vi "Calibration.vi"(7 "Show Front Panel":bool=TRUE, 8 "error in (no error)":errorcluster, 11 "file path (dialog if empty)":path=path "C:/Program Files/GE/Washer DOE/CalibrationDates.txt") -> (0 "error out":errorcluster, 3 "OutputData":string[][](array[string]))   [LabVIEW 2012]
uses:
  Calibration.ctl
  CalibrationTime.ctl
  Calibration_SN.ctl
  Equipment.vi
  <vilib>/Utility/file.llb/Write To Spreadsheet File (string).vi
panel:
  in  "Size":i32
  out "snta":string[](array[string])
  in  "Tab Control":enum32{"Calibration Dates", "File Location"}(tab)
  in  "Equipment Description":T1
  in  "Manufacturer":T1
  in  "Model Number":T1
  in  "Calibration ID":T1
  in  "Complete":bool
  out "concatenated string":string
  in  "Serial Number":T2
  in  "Last Calibrated":T3 {"Eq20" format="%<%x>T"; "Eq19" format="%<%x>T"; "Eq18" format="%<%x>T"; "Eq17" format="%<%x>T"; "Eq16" format="%<%x>T"; "Eq15" format="%<%x>T"; "Eq14" format="%<%x>T"; "Eq13" format="%<%x>T"; "Eq12" format="%<%x>T"; "Eq11" format="%<%x>T"; "Eq10" format="%<%x>T"; "Eq9" format="%<%x>T"; "Eq8" format="%<%x>T"; "Eq7" format="%<%x>T"; "Eq6" format="%<%x>T"; "Eq5" format="%<%x>T"; "Eq4" format="%<%x>T"; "Eq3" format="%<%x>T"; "Eq2" format="%<%x>T"; "Eq1" format="%<%x>T"}
  in  "Calibration Due":T3 {"Eq20" format="%<%x>T"; "Eq19" format="%<%x>T"; "Eq18" format="%<%x>T"; "Eq17" format="%<%x>T"; "Eq16" format="%<%x>T"; "Eq15" format="%<%x>T"; "Eq14" format="%<%x>T"; "Eq13" format="%<%x>T"; "Eq12" format="%<%x>T"; "Eq11" format="%<%x>T"; "Eq10" format="%<%x>T"; "Eq9" format="%<%x>T"; "Eq8" format="%<%x>T"; "Eq7" format="%<%x>T"; "Eq6" format="%<%x>T"; "Eq5" format="%<%x>T"; "Eq4" format="%<%x>T"; "Eq3" format="%<%x>T"; "Eq2" format="%<%x>T"; "Eq1" format="%<%x>T"}
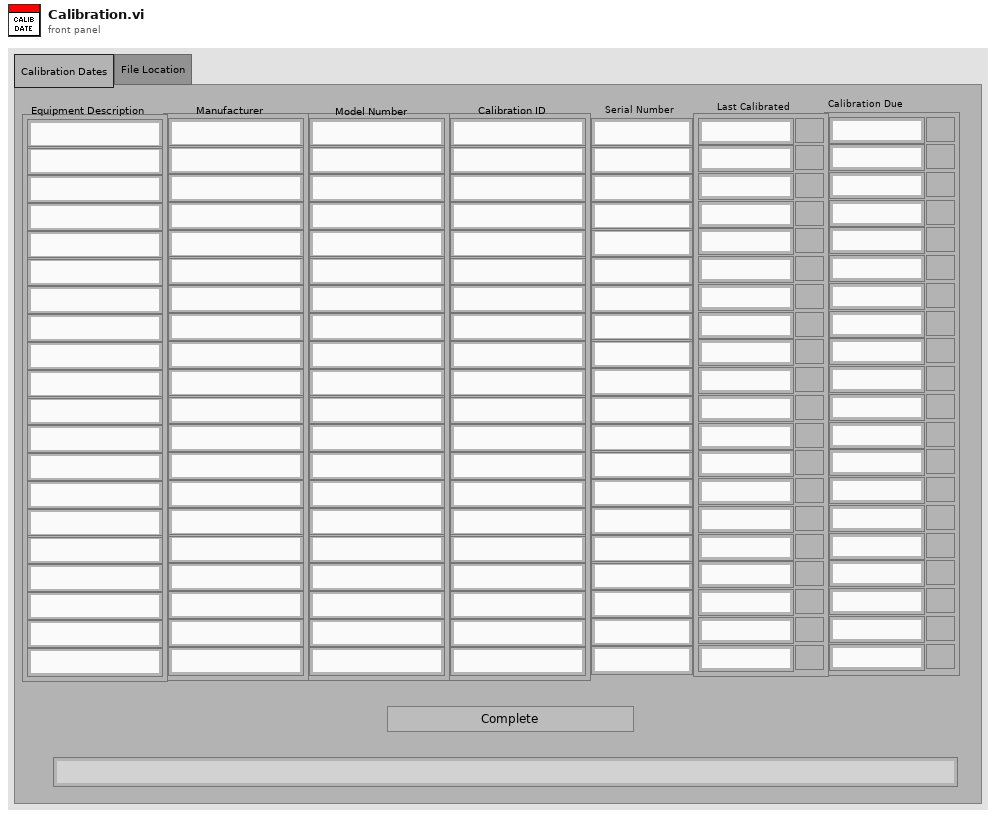
[diagram p1: front panel]
types:
  T1 = typedef "Calibration.ctl" = cluster{"Eq1":string, "Eq2":string, "Eq3":string, "Eq4":string, "Eq5":string, "Eq6":string, "Eq7":string, "Eq8":string, "Eq9":string, "Eq10":string, "Eq11":string, "Eq12":string, "Eq13":string, "Eq14":string, "Eq15":string, "Eq16":string, "Eq17":string, "Eq18":string, "Eq19":string, "Eq20":string}
  T2 = typedef "Calibration_SN.ctl" = cluster{"Eq1":string, "Eq2":string, "Eq3":string, "Eq4":string, "Eq5":string, "Eq6":string, "Eq7":string, "Eq8":string, "Eq9":string, "Eq10":string, "Eq11":string, "Eq12":string, "Eq13":string, "Eq14":string, "Eq15":string, "Eq16":string, "Eq17":string, "Eq18":string, "Eq19":string, "Eq20":string}
  T3 = typedef "CalibrationTime.ctl" = cluster{"Eq1":timestamp, "Eq2":timestamp, "Eq3":timestamp, "Eq4":timestamp, "Eq5":timestamp, "Eq6":timestamp, "Eq7":timestamp, "Eq8":timestamp, "Eq9":timestamp, "Eq10":timestamp, "Eq11":timestamp, "Eq12":timestamp, "Eq13":timestamp, "Eq14":timestamp, "Eq15":timestamp, "Eq16":timestamp, "Eq17":timestamp, "Eq18":timestamp, "Eq19":timestamp, "Eq20":timestamp}
  T4 = cluster{"Calibration Due":T3, "Last Calibrated":T3, "Serial Number":T2, "Calibration ID":T1, "Model Number":T1, "Manufacturer":T1, "Equipment Description":T1, i32}
  T5 = enum32{"invalid app kind", "Development System", "Run Time System", "Student Edition", "Embedded LabVIEW", "Evaluation", "Custom"}
  T6 = enum32{"Invalid", "Standard", "Closed", "Hidden", "Minimized", "Maximized"}
  T7 = cluster{"Core":cluster{"Current VI Reference":refnum<vi>, "Close Panel on Exit?":bool}, "Calibration Due":T3, "file path (dialog if empty)":path, "Serial Number":T2, "Calibration ID":T1, "Total Array":string[][], "Size":i32, "Last Calibrated":T3, "Model Number":T1, "Manufacturer":T1, "Equipment Description":T1}
  T8 = cluster{"Current VI Reference":refnum<vi>, "Close Panel on Exit?":bool}
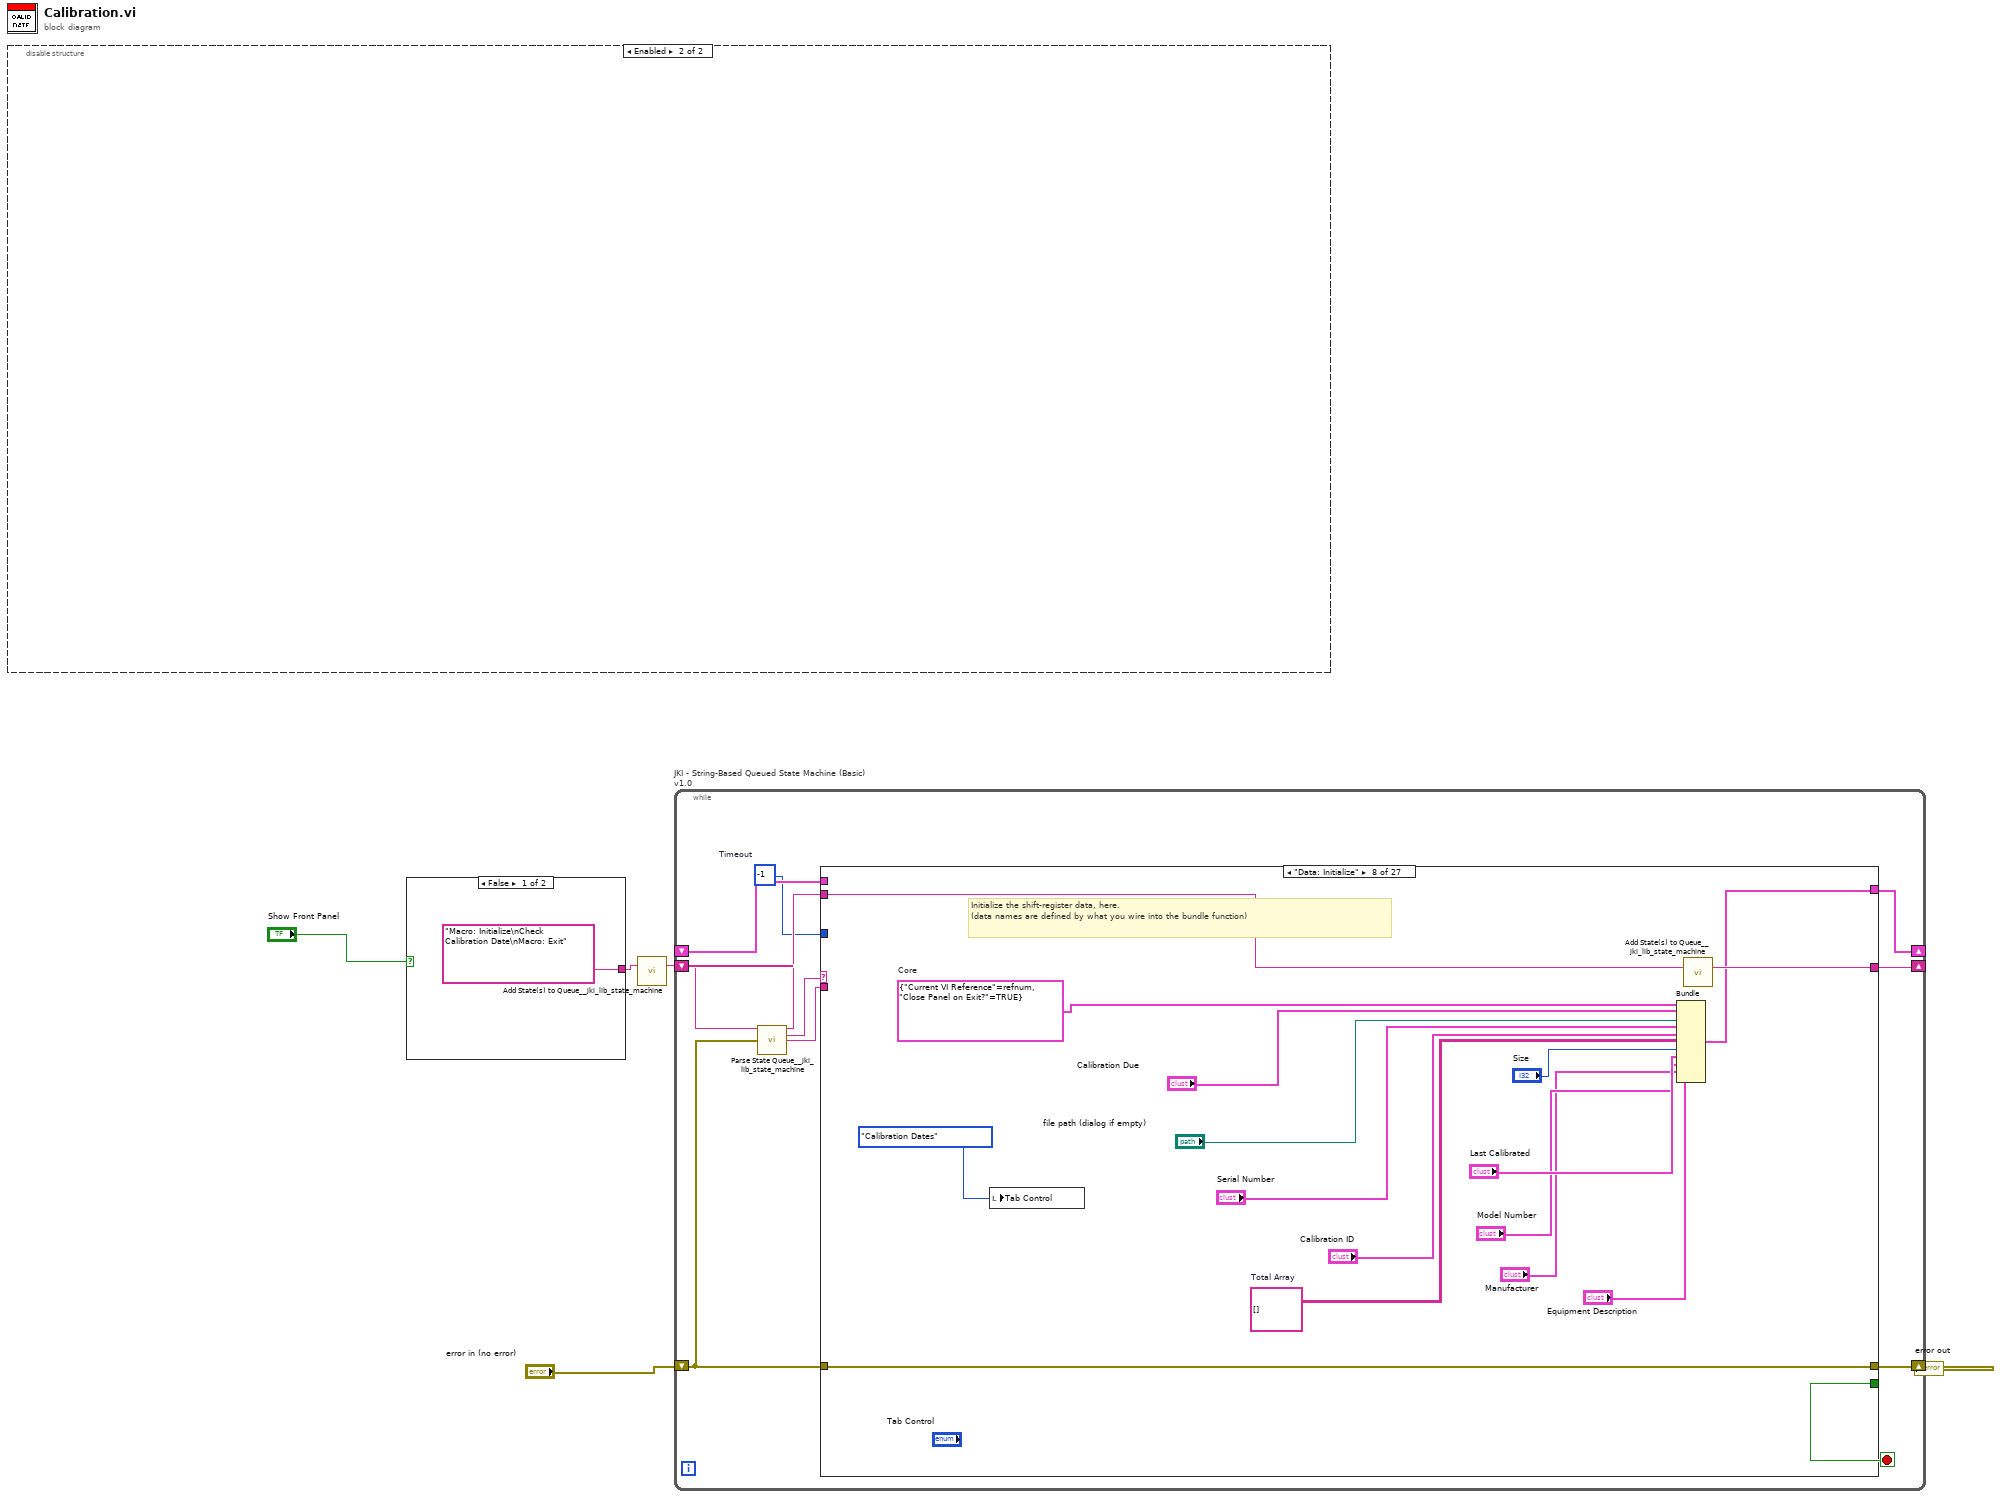
[diagram p0: block diagram]
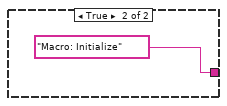
[diagram p2: hidden frame]
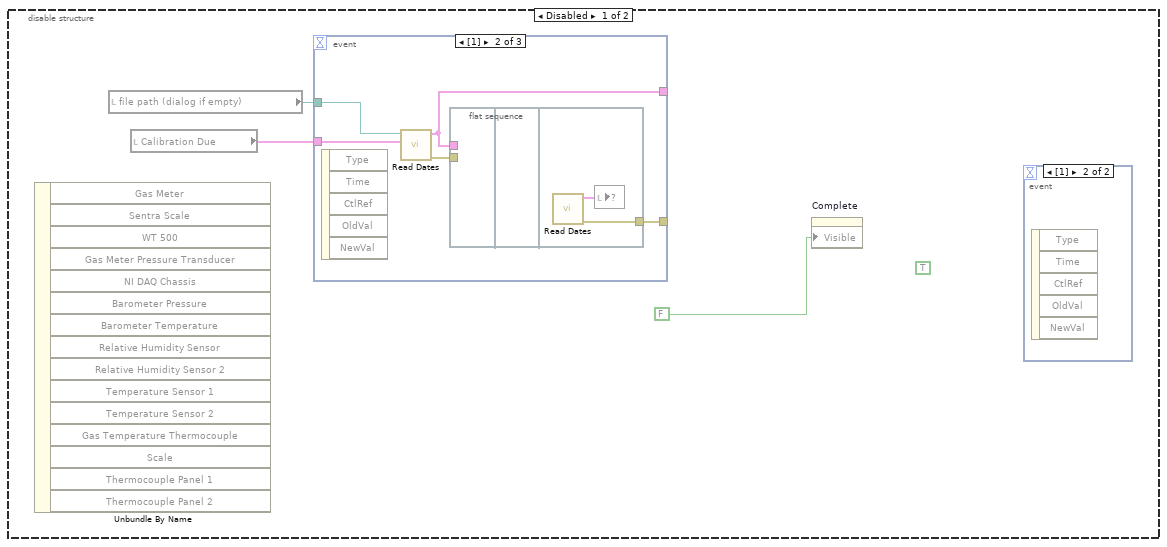
[diagram p3: hidden frame]
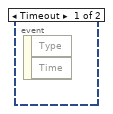
[diagram p4: hidden frame]
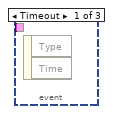
[diagram p5: hidden frame]
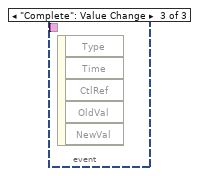
[diagram p6: hidden frame]
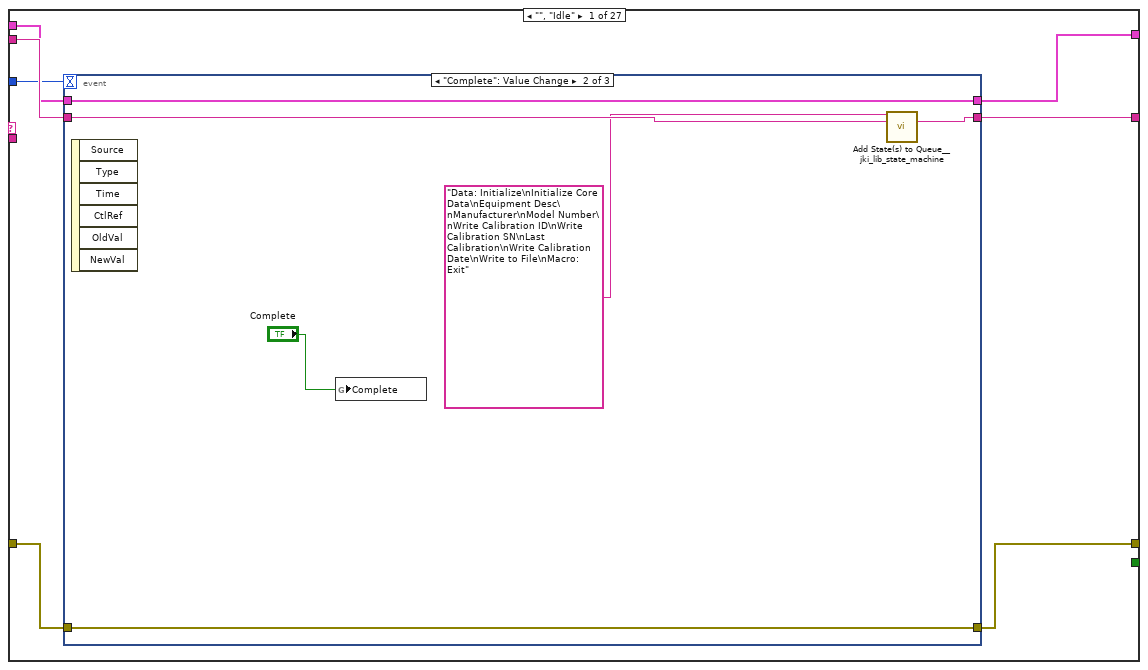
[diagram p7: hidden frame]
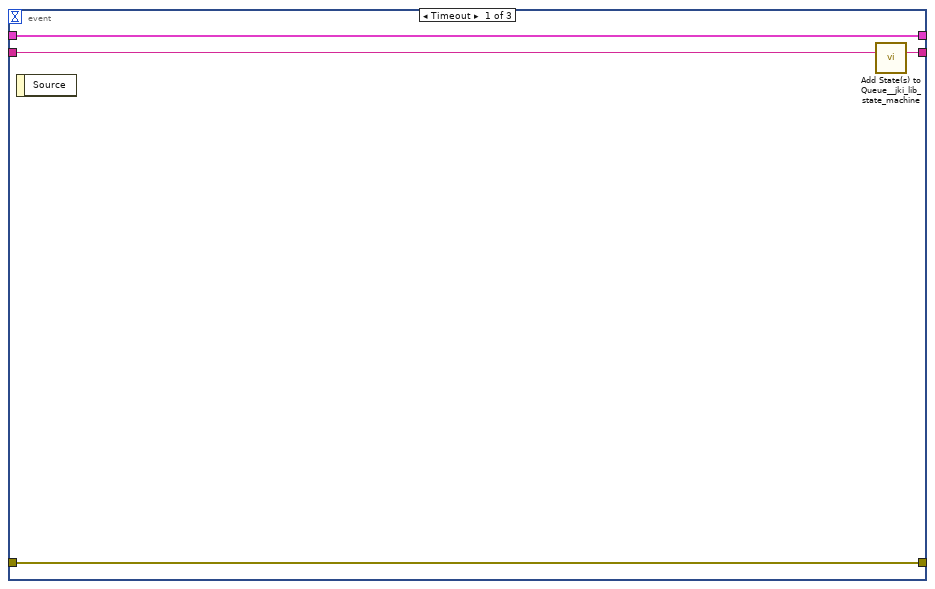
[diagram p8: hidden frame]
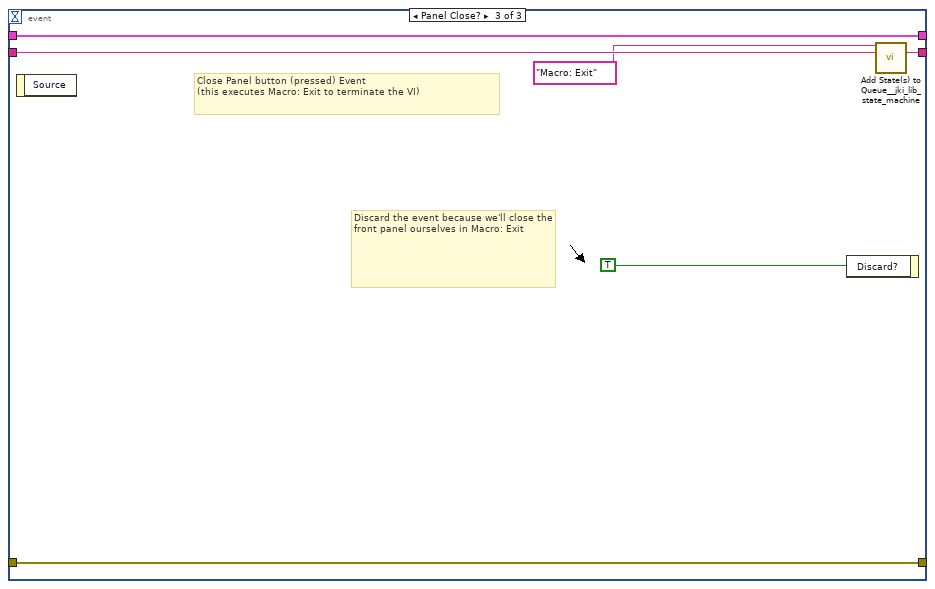
[diagram p9: hidden frame]
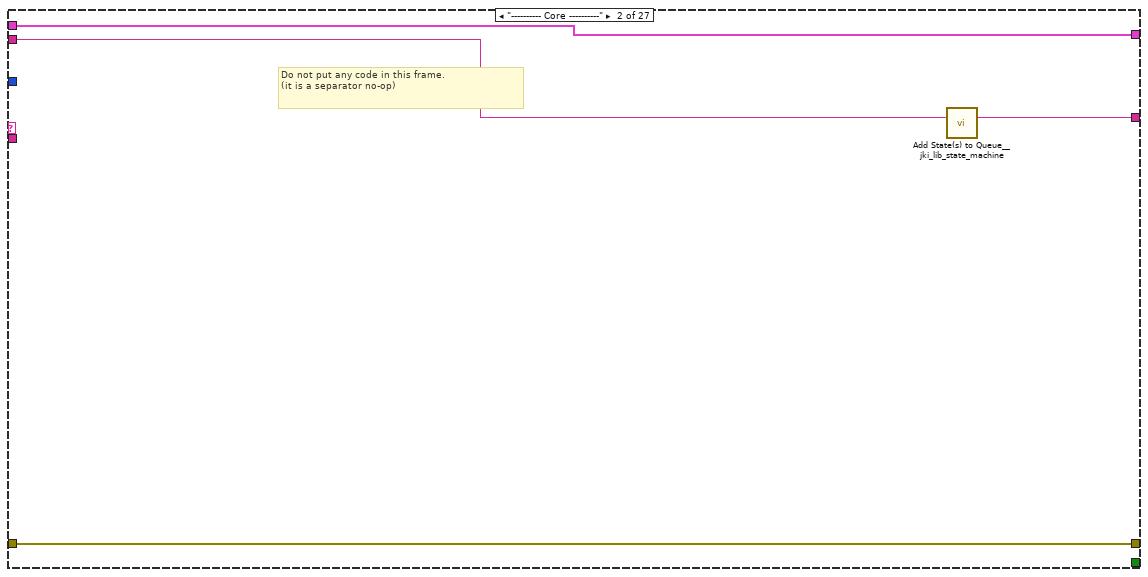
[diagram p10: hidden frame]
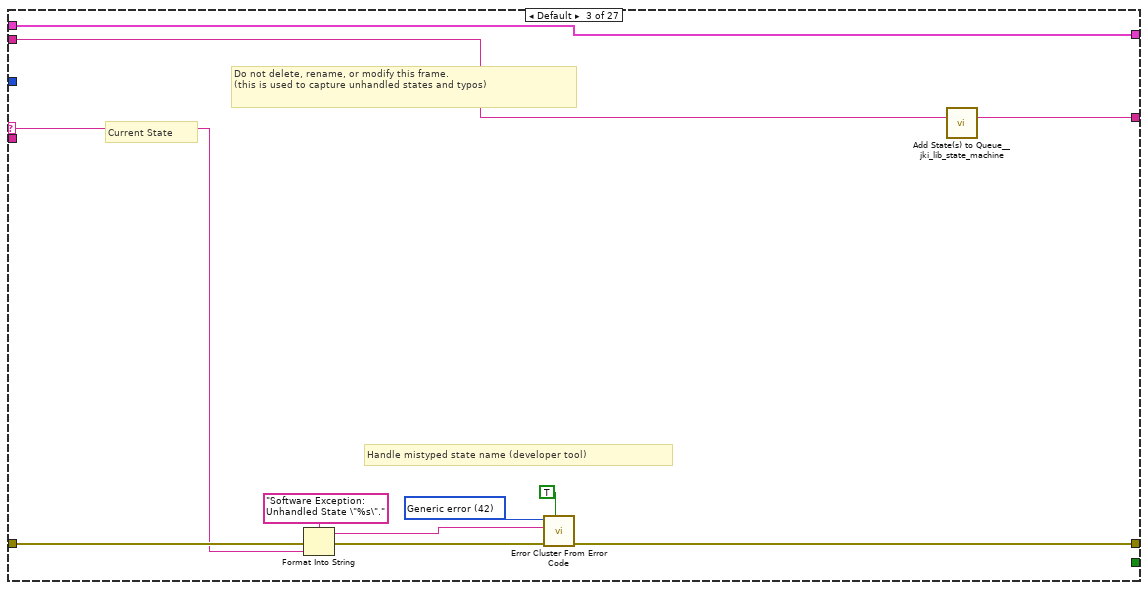
[diagram p11: hidden frame]
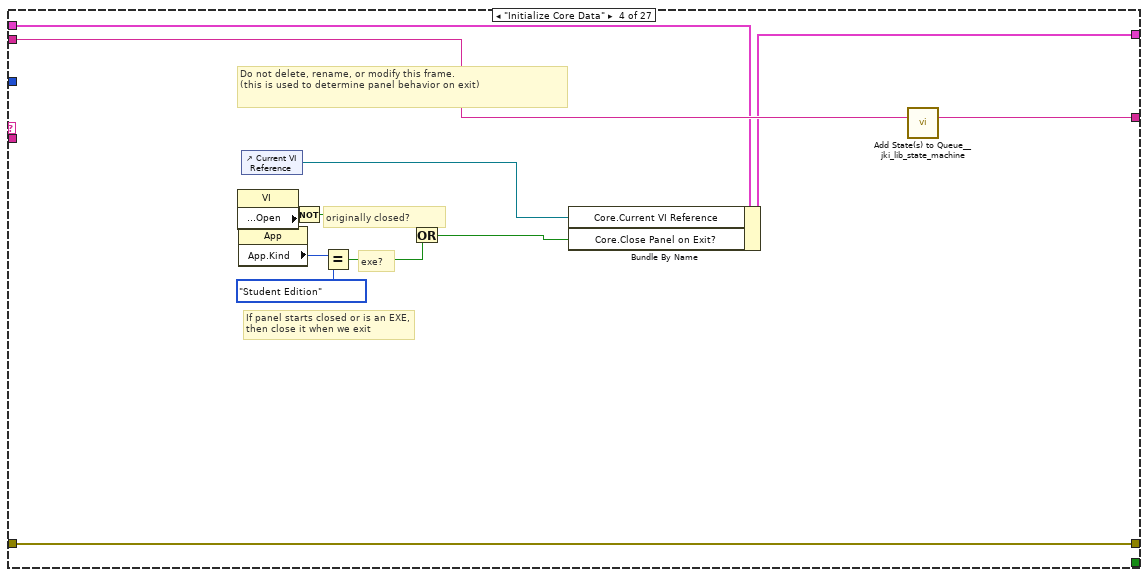
[diagram p12: hidden frame]
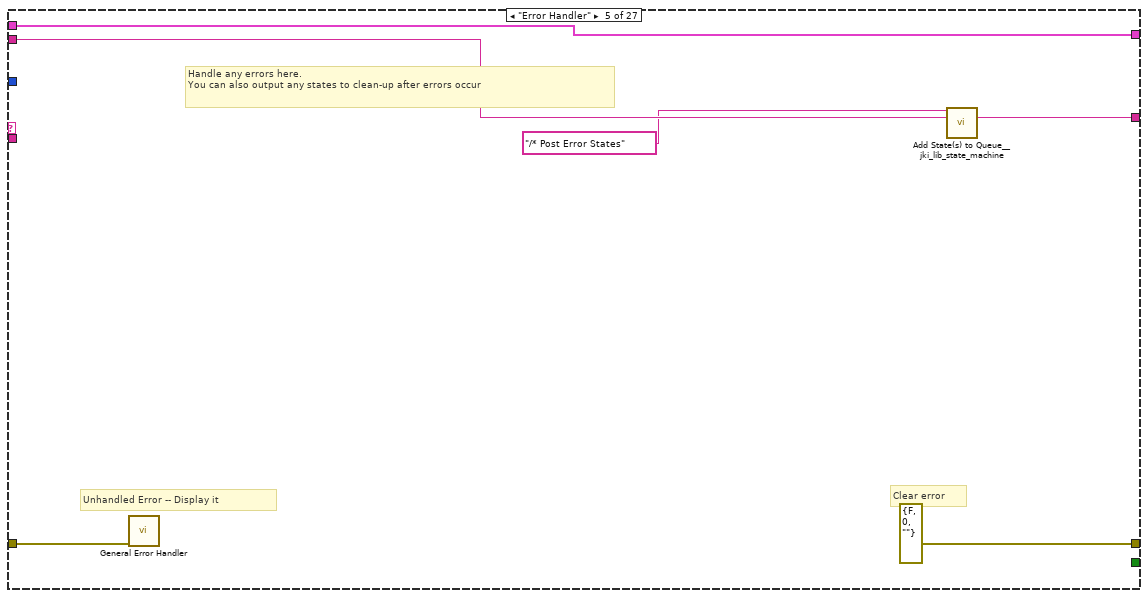
[diagram p13: hidden frame]
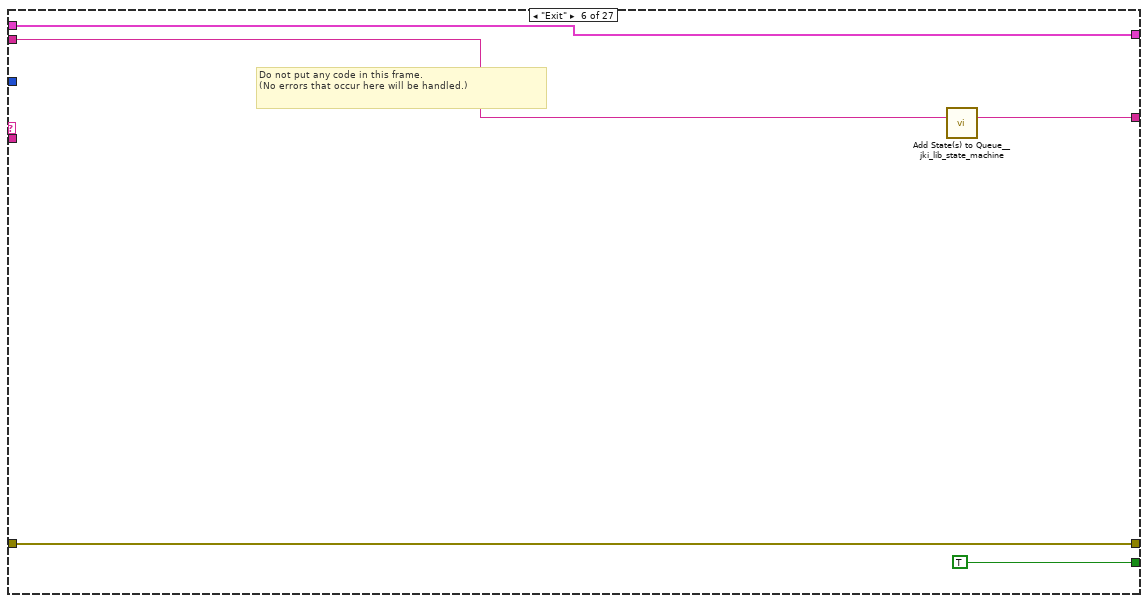
[diagram p14: hidden frame]
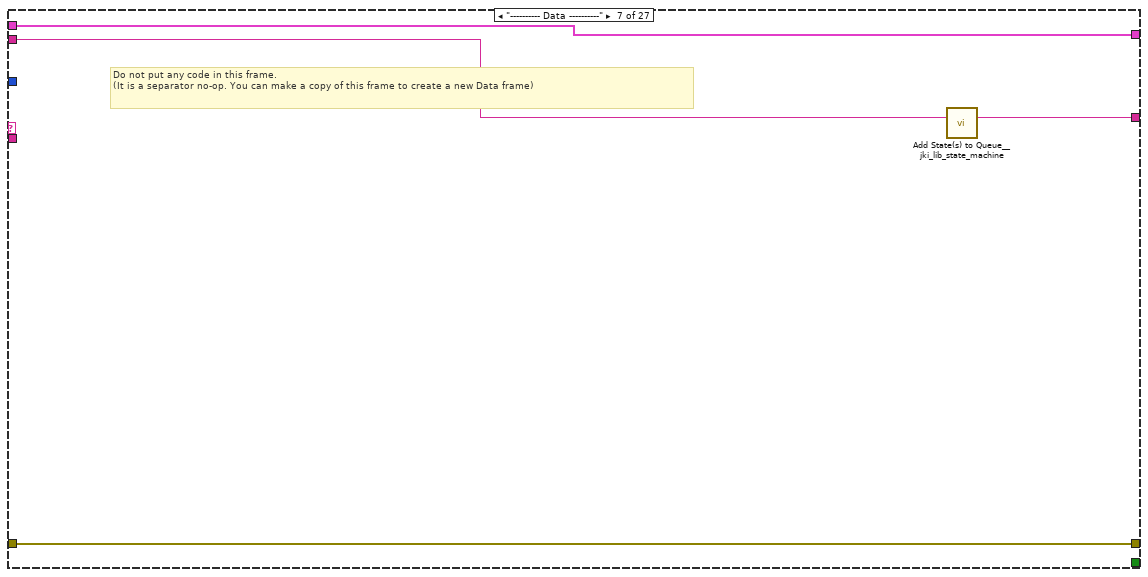
[diagram p15: hidden frame]
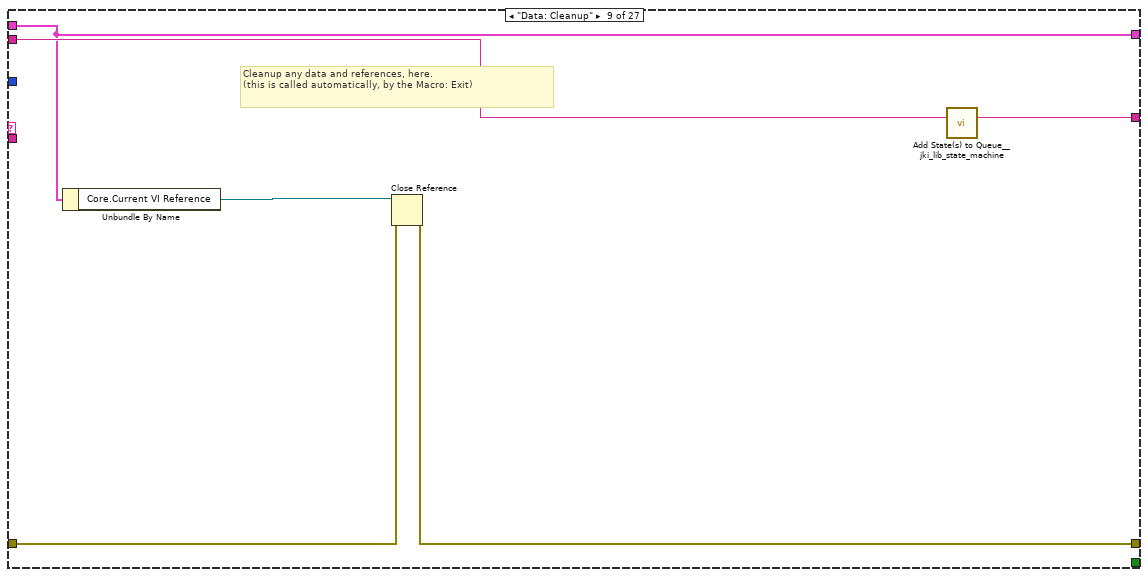
[diagram p16: hidden frame]
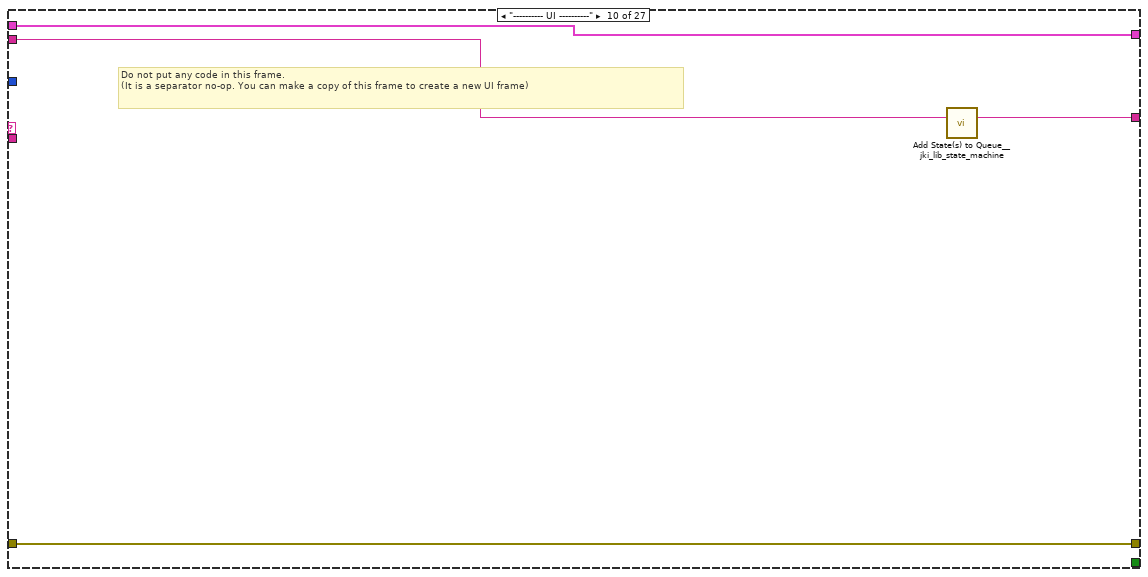
[diagram p17: hidden frame]
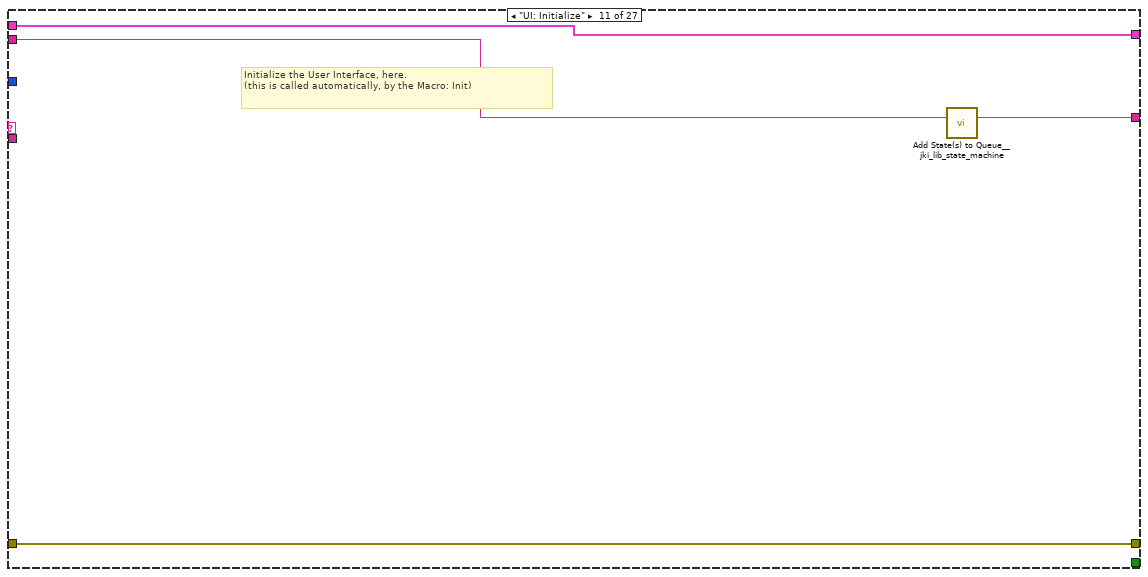
[diagram p18: hidden frame]
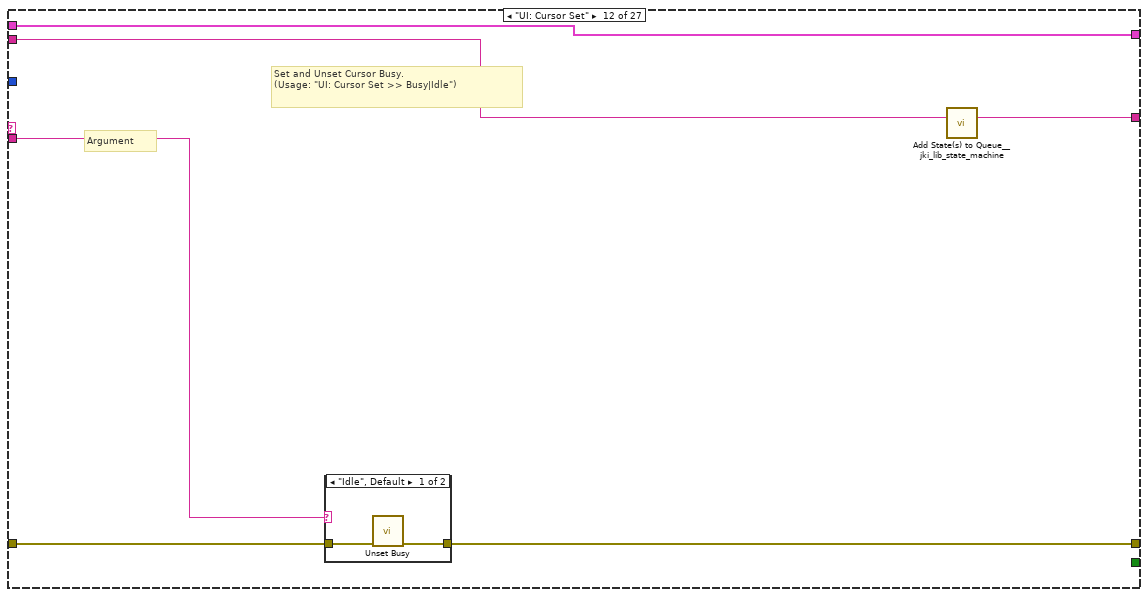
[diagram p19: hidden frame]
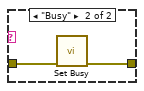
[diagram p20: hidden frame]
diagram:
  n1 = disable-structure shown="Enabled" {
    frame Disabled {
      w8 = TRUE ("Visible")
      n2 = Unbundle By Name() -> ()  [unwired: 1 in, 15 out]
      n3 = local read "file path (dialog if empty)"() -> (w6:path)
      n4 = local read "Calibration Due"() -> (w7:T3)
      n5 = event shown="[1]" {
        selector: _ -> [_ _ _]
        dyn-events: _ -> [_ _ _]
        timeout: _ -> [_ _ _]
        tunnel: [_ w12 _] -> _
        tunnel: [_ w15 _] -> _
        tunnel: w7 -> [_ w14 _]
        tunnel: w6 -> [_ w13 _]
        event Timeout {
          n6 = event-data() -> ()  [unwired: 1 in, 2 out]
        }
        event #1 (no event record) {
          n7 = event-data() -> ()  [unwired: 1 in, 5 out]
          n8 = call "Read Dates.vi"("Manufacturer"=w14, "Equipment Description"=w13) -> ("error out"=w11:errorcluster, "output cluster"=w12:T4)  [unwired: 8 in]
          n9 = flat-sequence {
            tunnel: w11 -> [_]
            tunnel: w12 -> [_]
            tunnel: [w16] -> w15
            frame #0 {
            }
            frame #1 {
            }
            frame #2 {
              n10 = call "Read Dates.vi"() -> ("error out"=w16:errorcluster, "output cluster"=w17:T4)  [unwired: 10 in]
              n11 = local write item#-1(w17) -> ()
            }
          }
        }
        event "Complete": Value Change {
          n12 = event-data() -> ()  [unwired: 1 in, 5 out]
        }
      }
      n13 = property on="Complete" class="Bool"("Visible"=FALSE) -> (error out=w9:errorcluster)  [unwired: 2 in, 1 out]
      n14 = event shown="[1]" {
        selector: _ -> [_ _]
        dyn-events: _ -> [_ _]
        timeout: _ -> [_ _]
        event Timeout {
          n15 = event-data() -> ()  [unwired: 1 in, 2 out]
        }
        event #1 (no event record) {
          n16 = event-data() -> ()  [unwired: 1 in, 5 out]
        }
      }
    }
    frame Enabled {
    }
  }
  n17 = case shown="False" "Show Front Panel" {
    tunnel: ["Macro: Initialize\nCheck Calibration Date\nMacro: Exit" "Macro: Initialize"] -> w4
    frame False {
    }
    frame True {
    }
  }
  n18 = call <vilib>:"Add State(s) to Queue__jki_lib_state_machine.vi"("State(s) in (\"\")"=w4) -> ("States Out"=w5:string)  [unwired: 14 in]
  n19 = while "JKI - String-Based Queued State Machine (Basic) v1.0" {
    shift-right: [w23] -> _
    shift-left: _ -> [w22]
    shift-right: [w26] -> w2
    shift-left: "error in (no error)" -> [w20]
    shift-right: [w25] -> _
    shift-left: w5 -> [w27]
    stop <- w24 stop-if-true
    w21 = -1  # Timeout
    n20 = call <vilib>:"Parse State Queue__jki_lib_state_machine.vi"("State Queue"=w27, "Error In (no error)"=w20) -> ("Remaining States"=w29:string, "Current State"=w30:string, "Arguments"=w28:string)  [unwired: 11 in]
    n21 = case shown="\"Data: Initialize\"" w30 {
      selector: w30 -> [_ _ w58 _ _ _ _ _ _ _ _ _ _ _ _ _ _ _ _ _ _ _ _ _ _ _ _]
      tunnel: w29 -> [w37 w57 w62 w80 w86 w91 w95 w111 w117 w121 w125 w131 w142 w168 w173 w183 w187 w209 w220 w361 w421 w481 w541 w601 w661 w743 w819]
      tunnel: w28 -> [_ _ _ _ _ _ _ _ _ _ _ w126 w136 _ _ _ _ _ _ _ _ _ _ _ _ _ _]
      tunnel: w22 -> [w35 w54 w60 w71 w83 w89 w92 _ w112 w118 w123 w129 w138 w165 w170 w180 w184 w207 w218 w355 w415 w475 w535 w595 w654 w736 w817]
      tunnel: [w34 w55 w64 w77 errorcluster {"status"=FALSE, "code"=0, "source"=""} ("error out") w88 w93 w108 w113 w119 w122 w127 w139 w166 w171 w181 w185 w204 w217 w356 w416 w476 w536 w596 w656 w738 w814] -> w26
      tunnel: w20 -> [w33 w55 w63 w77 w82 w88 w93 w108 w114 w119 w122 w128 w140 w166 w171 w181 w185 w205 w217 w357 w417 w477 w537 w597 w657 w739 w814]
      tunnel: [w36 w56 w61 w79 w85 w90 w94 w110 w116 w120 w124 w130 w141 w167 w172 w182 w186 w208 w219 w360 w420 w480 w540 w600 w660 w742 w818] -> w25
      tunnel: [_ _ _ _ _ TRUE _ _ _ _ _ _ _ _ _ _ _ _ _ _ _ _ _ _ _ _ _] -> w24
      tunnel: [w32 w54 w60 w78 w83 w89 w92 w109 w112 w118 w123 w129 w138 w165 w170 w180 w184 w206 w218 w354 w414 w474 w534 w594 w653 w735 w817] -> w23
      tunnel: w21 -> [w31 _ _ _ _ _ _ _ _ _ _ _ _ _ _ _ _ _ _ _ _ _ _ _ _ _ _]
      frame "", "Idle" {
        n22 = event shown="[1] \"Complete\": Value Change" {
          selector: _ -> [_ _ _]
          dyn-events: _ -> [_ _ _]
          timeout: w31 -> [_ _ _]
          tunnel: w37 -> [w41 w46 w53]
          tunnel: [w40 w47 w52] -> w36
          tunnel: w35 -> [w38 w43 w50]
          tunnel: [w39 w45 w51] -> w34
          tunnel: w33 -> [w39 w45 w51]
          tunnel: [w38 w43 w50] -> w32
          event Timeout {
            n23 = event-data() -> ()  [unwired: 1 in, 1 out]
            n24 = call <vilib>:"Add State(s) to Queue__jki_lib_state_machine.vi"("State(s) in (\"\")"=w41) -> ("States Out"=w40:string)  [unwired: 14 in]
          }
          event "Complete": Value Change {
            n25 = event-data() -> ()  [unwired: 1 in, 6 out]
            n26 = global write "Equipment.vi" "Complete"("Complete") -> ()
            n27 = call <vilib>:"Add State(s) to Queue__jki_lib_state_machine.vi"("State(s) in Front (\"\")"="Data: Initialize\nInitialize Core Data\nEquipment Desc\nManufacturer\nModel Number\nWrite Calibration ID\nWrite Calibration SN\nLast Calibration\nWrite Calibration Date\nWrite to File\nMacro: Exit", "State(s) in (\"\")"=w46) -> ("States Out"=w47:string)  [unwired: 13 in]
          }
          event Panel Close? {
            # "Discard the event because we'll close the front panel ourselves in Macro: Exit"
            # "Close Panel button (pressed) Event\n(this executes Macro: Exit to terminate the VI)"
            n28 = event-data() -> ()  [unwired: 1 in, 1 out]
            n29 = event-data("Discard?"=TRUE) -> ()  [unwired: 1 in, 1 out]
            n30 = call <vilib>:"Add State(s) to Queue__jki_lib_state_machine.vi"("State(s) in Front (\"\")"="Macro: Exit", "State(s) in (\"\")"=w53) -> ("States Out"=w52:string)  [unwired: 13 in]
          }
        }
      }
      frame "---------- Core ----------" {
        # "Do not put any code in this frame.\n(it is a separator no-op)"
        n31 = call <vilib>:"Add State(s) to Queue__jki_lib_state_machine.vi"("State(s) in (\"\")"=w57) -> ("States Out"=w56:string)  [unwired: 14 in]
      }
      frame Default {
        w67 = 42 items=["No error", "Argument error", "Memory is full", "Out of zone", "End of file", "File already open", "Generic file I/O error", "File not found", "File permission error", "Disk is full", "Duplicate path", "Too many files open", "System feature not enabled", "Resource file not found", "Cannot add resource", "Resource not found", "Image not found", "Image memory error", "Pen does not exist", "Config type invalid", "Config token not found", "Config parse error", "Config memory error", "Bad external code format", "Bad external code offset", "External code not present", "Null window", "Destroy window error", "Null menu", "Print aborted", "Bad print record", "Print driver error", "Windows error during printing", "Memory error during printing", "Print dialog error", "Generic print error", "Invalid device refnum", "Device not found", "Device parameter error", "Device unit error", "Cannot open device", "Device call aborted", "Generic error", "Cancelled by user", "Object ID too low", "Object ID too high", "Object not in heap", "Unknown heap", "Unknown object (invalid DefProc)", "Unknown object (DefProc not in table)", "Message out of range", "Invalid (null) method", "Unknown message", "Manager call not supported", "Bad address", "Network operation in progress", "Network operation timed out", "Connection is busy", "Network attribute not supported", "Network error", "Address in use", "System out of memory", "Connection aborted", "Connection refused", "Not connected", "Already connected", "Connection closed", "Initialization error (interapplication manager)", "Bad occurrence", "Wait on unbound occurrence handler", "Occurrence queue overflow", "Datalog type conflict", "Unused", "Unrecognized type (interapplication manager)", "Memory corrupt", "Failed to make temporary DLL", "Old CIN version", "Drag socket not found", "Failed to load drop-object", "Failed to register OLE object", "Failed to release OLE object", "Format specifier type mismatch", "Unknown format specifier", "Too few format specifiers", "Too many format specifiers", "Scan failed", "Newer CIN version", "Error converting to variant", "Runtime menu error", "Password tampered", "Variant attribute not found", "Incompatible variant data type", "Event data is not available", "Event Store is not present", "Occurrence is not found", "Event Queue is not created", "Event info is not available", "Refnum passed is NULL", "Error retrieving Class GUID", "Error retrieving CoClass GUID", "Error retrieving TypeLib GUID.", "Bad built application magic bytes.", "Specific driver is different from the specific driver associated with the Logical Name.", "There is no session opened to the class driver.", "Max Error", "MAX - Error with config objects", "MAX - Error loading configuration", "MAX - Group not supported"]
        # "Current State"
        # "Do not delete, rename, or modify this frame.\n(this is used to capture unhandled states and typos)"
        # "Handle mistyped state name (developer tool)"
        n32 = Format Into String(format string="Software Exception: Unhandled State \"%s\"." ("message"), error in=w63, w58) -> (resulting string=w66:string, error out=w65:errorcluster)  [unwired: 1 in]
        n33 = call <vilib>:"Error Cluster From Error Code.vi"("show call chain? (False)"=TRUE, "error in (no error)"=w65, "error message (\"\")"=w66, "error code (0)"=w67) -> ("error out"=w64:errorcluster)  [unwired: 5 in]
        n34 = call <vilib>:"Add State(s) to Queue__jki_lib_state_machine.vi"("State(s) in (\"\")"=w62) -> ("States Out"=w61:string)  [unwired: 14 in]
      }
      frame "Initialize Core Data" {
        # "Do not delete, rename, or modify this frame.\n(this is used to determine panel behavior on exit)"
        # "originally closed?"
        # "exe?"
        # "If panel starts closed or is an EXE, then close it when we exit"
        n35 = property class="VI"() -> ("Front Panel.Open"=w76:bool)  [unwired: 2 in, 2 out]
        n36 = property class="App"() -> ("App.Kind"=w75:T5)  [unwired: 2 in, 2 out]
        n37 = control-ref of="Current VI Reference"() -> (w69:refnum<vi>)
        n38 = Not(x=w76) -> (.not. x?=w73:bool)
        n39 = Equal?(x=w75, y=T5."Student Edition" ("Application:Kind")) -> (x = y?=w72:bool)
        n40 = Or(x=w73, y=w72) -> (x .or. y?=w70:bool)
        n41 = Bundle By Name(cluster=w71, "Core.Current VI Reference"=w69, "Core.Close Panel on Exit?"=w70) -> (w78:T7)
        n42 = call <vilib>:"Add State(s) to Queue__jki_lib_state_machine.vi"("State(s) in (\"\")"=w80) -> ("States Out"=w79:string)  [unwired: 14 in]
      }
      frame "Error Handler" {
        # "Unhandled Error -- Display it"
        # "Handle any errors here.\nYou can also output any states to clean-up after errors occur"
        # "Clear error"
        n43 = call <vilib>:"General Error Handler.vi"("error in (no error)"=w82) -> ()  [unwired: 10 in, 5 out]
        n44 = call <vilib>:"Add State(s) to Queue__jki_lib_state_machine.vi"("State(s) in Front (\"\")"="/* Post Error States", "State(s) in (\"\")"=w86) -> ("States Out"=w85:string)  [unwired: 13 in]
      }
      frame "Exit" {
        # "Do not put any code in this frame.\n(No errors that occur here will be handled.)"
        n45 = call <vilib>:"Add State(s) to Queue__jki_lib_state_machine.vi"("State(s) in (\"\")"=w91) -> ("States Out"=w90:string)  [unwired: 14 in]
      }
      frame "---------- Data ----------" {
        # "Do not put any code in this frame.\n(It is a separator no-op. You can make a copy of this frame to create a new Data frame)"
        n46 = call <vilib>:"Add State(s) to Queue__jki_lib_state_machine.vi"("State(s) in (\"\")"=w95) -> ("States Out"=w94:string)  [unwired: 14 in]
      }
      frame "Data: Initialize" {
        w105 = string[][] []  # Total Array
        w107 = T8 {"Current VI Reference"=refnum, "Close Panel on Exit?"=TRUE}  # Core
        # "Initialize the shift-register data, here.\n(data names are defined by what you wire into the bundle function)"
        n47 = local write "Tab Control"(enum32{"Calibration Dates", "File Location"}."Calibration Dates" ("Tab Control")) -> ()
        n48 = Bundle("Core"=w107, "Calibration Due"="Calibration Due", "file path (dialog if empty)"="file path (dialog if empty)", "Serial Number"="Serial Number", "Calibration ID"="Calibration ID", "Total Array"=w105, "Size"="Size", "Last Calibrated"="Last Calibrated", "Model Number"="Model Number", "Manufacturer"="Manufacturer", "Equipment Description"="Equipment Description") -> (w109:T7)  [unwired: 1 in]
        n49 = call <vilib>:"Add State(s) to Queue__jki_lib_state_machine.vi"("State(s) in (\"\")"=w111) -> ("States Out"=w110:string)  [unwired: 14 in]
      }
      frame "Data: Cleanup" {
        # "Cleanup any data and references, here.\n(this is called automatically, by the Macro: Exit)"
        n50 = Unbundle By Name(w112) -> ("Core.Current VI Reference"=w115:refnum<vi>)
        n51 = Close Reference(reference=w115, error in (no error)=w114) -> (error out=w113:errorcluster)
        n52 = call <vilib>:"Add State(s) to Queue__jki_lib_state_machine.vi"("State(s) in (\"\")"=w117) -> ("States Out"=w116:string)  [unwired: 14 in]
      }
      frame "---------- UI ----------" {
        # "Do not put any code in this frame.\n(It is a separator no-op. You can make a copy of this frame to create a new UI frame)"
        n53 = call <vilib>:"Add State(s) to Queue__jki_lib_state_machine.vi"("State(s) in (\"\")"=w121) -> ("States Out"=w120:string)  [unwired: 14 in]
      }
      frame "UI: Initialize" {
        # "Initialize the User Interface, here.\n(this is called automatically, by the Macro: Init)"
        n54 = call <vilib>:"Add State(s) to Queue__jki_lib_state_machine.vi"("State(s) in (\"\")"=w125) -> ("States Out"=w124:string)  [unwired: 14 in]
      }
      frame "UI: Cursor Set" {
        # "Argument"
        # "Set and Unset Cursor Busy.\n(Usage: \"UI: Cursor Set >> Busy|Idle\")"
        n55 = case shown="\"Idle\", Default" w126 {
          tunnel: w128 -> [w133 w135]
          tunnel: [w132 w134] -> w127
          frame "Idle", Default {
            n56 = call <vilib>:"Unset Busy.vi"("error in (no error)"=w133) -> ("error out"=w132:errorcluster)  [unwired: 10 in]
          }
          frame "Busy" {
            n57 = call <vilib>:"Set Busy.vi"("error in (no error)"=w135) -> ("error out"=w134:errorcluster)  [unwired: 9 in, 1 out]
          }
        }
        n58 = call <vilib>:"Add State(s) to Queue__jki_lib_state_machine.vi"("State(s) in (\"\")"=w131) -> ("States Out"=w130:string)  [unwired: 14 in]
      }
      frame "UI: Front Panel State" {
        # "Argument"
        # "Set Front Panel Open or Closed\n(Usage: \"UI: Front Panel State >> Open|Close\")"
        n59 = Unbundle By Name(w138) -> ("Core.Current VI Reference"=w137:refnum<vi>)
        n60 = case shown="\"Open\", Default" w136 {
          tunnel: w140 -> [w146 w159]
          tunnel: [w148 w160] -> w139
          tunnel: w137 -> [w147 w157]
          frame "Open", Default {
            n61 = property class="VI"(reference=w147, error in=w146) -> (reference out=w144:refnum<vi>, error out=w145:errorcluster, "Front Panel.Open"=w143:bool)
            n62 = case shown="True" w143 {
              tunnel: [w151 w154] -> w148
              tunnel: w145 -> [w150 w154]
              tunnel: w144 -> [w149 _]
              frame False {
                n63 = invoke class="VI" method="FP.Open"(reference=w149, error in=w150, "Activate"=TRUE, "State"=T6."Standard") -> (error out=w151:errorcluster)  [unwired: 1 in, 4 out]
              }
              frame True {
              }
            }
          }
          frame "Close" {
            n64 = property class="VI"(reference=w157, error in=w159) -> (reference out=w156:refnum<vi>, error out=w158:errorcluster, "Front Panel.Open"=w155:bool)
            n65 = case shown="True" w155 {
              tunnel: [w161 w164] -> w160
              tunnel: w158 -> [w161 w163]
              tunnel: w156 -> [_ w162]
              frame False {
              }
              frame True {
                n66 = invoke class="VI" method="FP.Close"(reference=w162, error in=w163) -> (error out=w164:errorcluster)  [unwired: 1 in, 2 out]
              }
            }
          }
        }
        n67 = call <vilib>:"Add State(s) to Queue__jki_lib_state_machine.vi"("State(s) in (\"\")"=w142) -> ("States Out"=w141:string)  [unwired: 14 in]
      }
      frame "---------- Macro ----------" {
        # "Do not put any code in this frame.\n(It is a separator no-op. You can make a copy of this frame to create a new Macro frame)"
        n68 = call <vilib>:"Add State(s) to Queue__jki_lib_state_machine.vi"("State(s) in (\"\")"=w168) -> ("States Out"=w167:string)  [unwired: 14 in]
      }
      frame "Macro: Initialize" {
        w169 = "Data: Initialize\nInitialize Core Data\nUI: Initialize\nUI: Front Panel State >> Open\nRead\nCheck Calibration Date"  # Data: Initialize Initialize Core Data UI: Initialize UI: Front Panel State >> Open Read Check Calibration Date
        # "Initialization Macro\n(This is called once, when the VI starts)"
        n69 = call <vilib>:"Add State(s) to Queue__jki_lib_state_machine.vi"("State(s) in Front (\"\")"=w169, "State(s) in (\"\")"=w173) -> ("States Out"=w172:string)  [unwired: 13 in]
      }
      frame "Macro: Exit" {
        # "Exit Macro\n(This is called once, when the VI exits)"
        n70 = Unbundle By Name(w180) -> ("Core.Close Panel on Exit?"=w179:bool)
        n71 = Select(t="UI: Front Panel State >> Close", s=w179, f="") -> (s? t:f=w176:string)
        n72 = call <vilib>:"Add State(s) to Queue__jki_lib_state_machine.vi"("State(s) in (\"\")"=w176, "State(s) at Back (\"\")"="Data: Cleanup\nExit") -> ("States Out"=w174:string)  [unwired: 13 in]
        n73 = call <vilib>:"Add State(s) to Queue__jki_lib_state_machine.vi"("State(s) in Front (\"\")"=w174, "State(s) in (\"\")"=w183) -> ("States Out"=w182:string)  [unwired: 13 in]
      }
      frame "---------- New Category ----------" {
        # "Template Separator\n(You can make a copy of, or modify, this frame)"
        n74 = call <vilib>:"Add State(s) to Queue__jki_lib_state_machine.vi"("State(s) in (\"\")"=w187) -> ("States Out"=w186:string)  [unwired: 14 in]
      }
      frame "Read" {
        n75 = Unbundle By Name(w207) -> ("file path (dialog if empty)"=w196:path, "Equipment Description"=w203:T1, "Manufacturer"=w202:T1, "Model Number"=w201:T1, "Calibration ID"=w200:T1, "Serial Number"=w199:T2, "Last Calibrated"=w198:T3, "Calibration Due"=w197:T3)
        n76 = call "Read Dates.vi"("File Path"=w196, "Calibration Due"=w197, "Last Calibrated"=w198, "Serial Number"=w199, "Calibration ID"=w200, "error in (no error)"=w205, "Model Number"=w201, "Manufacturer"=w202, "Equipment Description"=w203) -> ("error out"=w204:errorcluster, "output cluster"=w195:T4)  [unwired: 1 in]
        n77 = Unbundle By Name(w195) -> ("Equipment Description"=w191:T1, "Manufacturer"=w190:T1, "Model Number"=w189:T1, "Calibration ID"=w192:T1, "Serial Number"=w193:T2, "Last Calibrated"=w188:T3, "Calibration Due"=w194:T3)
        n78 = property on="Calibration ID" class="Clust (strict)"("Value"=w192) -> ()  [unwired: 2 in, 2 out]
        n79 = property on="Serial Number" class="Clust (strict)"("Value"=w193) -> ()  [unwired: 2 in, 2 out]
        n80 = property on="Last Calibrated" class="Clust (strict)"("Value"=w188) -> ()  [unwired: 2 in, 2 out]
        n81 = property on="Calibration Due" class="Clust (strict)"("Value"=w194) -> ()  [unwired: 2 in, 2 out]
        n82 = Bundle By Name(cluster=w207, "Equipment Description"=w191, "Manufacturer"=w190, "Model Number"=w189, "Calibration ID"=w192, "Serial Number"=w193, "Last Calibrated"=w188, "Calibration Due"=w194) -> (w206:T7)
        n83 = property on="Equipment Description" class="Clust (strict)"("Value"=w191) -> ()  [unwired: 2 in, 2 out]
        n84 = property on="Manufacturer" class="Clust (strict)"("Value"=w190) -> ()  [unwired: 2 in, 2 out]
        n85 = property on="Model Number" class="Clust (strict)"("Value"=w189) -> ()  [unwired: 2 in, 2 out]
        n86 = call <vilib>:"Add State(s) to Queue__jki_lib_state_machine.vi"("State(s) in (\"\")"=w209) -> ("States Out"=w208:string)  [unwired: 14 in]
      }
      frame "Check Calibration Date" {
        # "Your code here.\n(You can make a copy of, or modify, this frame)"
        n87 = Unbundle By Name(w218) -> ("Calibration Due"=w216:T3, "Size"=w215:i32)  [unwired: 1 out]
        n88 = for {
          N: w215 -> [_]
          tunnel: w216 -> [w227]
          tunnel: [w225] -> w214 mode=indexing
          i -> [w226]
          n89 = case shown="0, Default" w226 {
            tunnel: w227 -> [w233 w239 w245 w251 w257 w263 w269 w275 w281 w287 w293 w299 w305 w311 w317 w323 w329 w335 w341 w347]
            tunnel: [w228 w234 w240 w246 w252 w258 w264 w270 w276 w282 w288 w294 w300 w306 w312 w318 w324 w330 w336 w342] -> w225
            frame 0, Default {
              n90 = Get Date/Time In Seconds() -> (seconds since 1Jan1904=w232:timestamp)
              n91 = Unbundle By Name(w233) -> ("Eq1"=w231:timestamp)
              n92 = Get Date/Time String(seconds (now)=w232) -> (date string=w229:string)  [unwired: 2 in, 1 out]
              n93 = Get Date/Time String(seconds (now)=w231) -> (date string=w230:string)  [unwired: 2 in, 1 out]
              n94 = call "DateString-Days.vi"("First date"=w229, "Second date"=w230) -> ("Elapsed days"=w228:i32)  [unwired: 8 in, 1 out]
            }
            frame 1 {
              n95 = Unbundle By Name(w239) -> ("Eq2"=w235:timestamp)
              n96 = Get Date/Time In Seconds() -> (seconds since 1Jan1904=w238:timestamp)
              n97 = Get Date/Time String(seconds (now)=w238) -> (date string=w236:string)  [unwired: 2 in, 1 out]
              n98 = Get Date/Time String(seconds (now)=w235) -> (date string=w237:string)  [unwired: 2 in, 1 out]
              n99 = call "DateString-Days.vi"("First date"=w236, "Second date"=w237) -> ("Elapsed days"=w234:i32)  [unwired: 8 in, 1 out]
            }
            frame 2 {
              n100 = Get Date/Time In Seconds() -> (seconds since 1Jan1904=w244:timestamp)
              n101 = Unbundle By Name(w245) -> ("Eq3"=w241:timestamp)
              n102 = Get Date/Time String(seconds (now)=w244) -> (date string=w242:string)  [unwired: 2 in, 1 out]
              n103 = Get Date/Time String(seconds (now)=w241) -> (date string=w243:string)  [unwired: 2 in, 1 out]
              n104 = call "DateString-Days.vi"("First date"=w242, "Second date"=w243) -> ("Elapsed days"=w240:i32)  [unwired: 8 in, 1 out]
            }
            frame 3 {
              n105 = Get Date/Time In Seconds() -> (seconds since 1Jan1904=w250:timestamp)
              n106 = Unbundle By Name(w251) -> ("Eq4"=w247:timestamp)
              n107 = Get Date/Time String(seconds (now)=w250) -> (date string=w248:string)  [unwired: 2 in, 1 out]
              n108 = Get Date/Time String(seconds (now)=w247) -> (date string=w249:string)  [unwired: 2 in, 1 out]
              n109 = call "DateString-Days.vi"("First date"=w248, "Second date"=w249) -> ("Elapsed days"=w246:i32)  [unwired: 8 in, 1 out]
            }
            frame 4 {
              n110 = Get Date/Time In Seconds() -> (seconds since 1Jan1904=w256:timestamp)
              n111 = Unbundle By Name(w257) -> ("Eq5"=w253:timestamp)
              n112 = Get Date/Time String(seconds (now)=w256) -> (date string=w254:string)  [unwired: 2 in, 1 out]
              n113 = Get Date/Time String(seconds (now)=w253) -> (date string=w255:string)  [unwired: 2 in, 1 out]
              n114 = call "DateString-Days.vi"("First date"=w254, "Second date"=w255) -> ("Elapsed days"=w252:i32)  [unwired: 8 in, 1 out]
            }
            frame 5 {
              n115 = Get Date/Time In Seconds() -> (seconds since 1Jan1904=w262:timestamp)
              n116 = Unbundle By Name(w263) -> ("Eq6"=w259:timestamp)
              n117 = Get Date/Time String(seconds (now)=w262) -> (date string=w260:string)  [unwired: 2 in, 1 out]
              n118 = Get Date/Time String(seconds (now)=w259) -> (date string=w261:string)  [unwired: 2 in, 1 out]
              n119 = call "DateString-Days.vi"("First date"=w260, "Second date"=w261) -> ("Elapsed days"=w258:i32)  [unwired: 8 in, 1 out]
            }
            frame 6 {
              n120 = Get Date/Time In Seconds() -> (seconds since 1Jan1904=w268:timestamp)
              n121 = Unbundle By Name(w269) -> ("Eq7"=w265:timestamp)
              n122 = Get Date/Time String(seconds (now)=w268) -> (date string=w266:string)  [unwired: 2 in, 1 out]
              n123 = Get Date/Time String(seconds (now)=w265) -> (date string=w267:string)  [unwired: 2 in, 1 out]
              n124 = call "DateString-Days.vi"("First date"=w266, "Second date"=w267) -> ("Elapsed days"=w264:i32)  [unwired: 8 in, 1 out]
            }
            frame 7 {
              n125 = Get Date/Time In Seconds() -> (seconds since 1Jan1904=w274:timestamp)
              n126 = Get Date/Time String(seconds (now)=w274) -> (date string=w272:string)  [unwired: 2 in, 1 out]
              n127 = Unbundle By Name(w275) -> ("Eq8"=w271:timestamp)
              n128 = Get Date/Time String(seconds (now)=w271) -> (date string=w273:string)  [unwired: 2 in, 1 out]
              n129 = call "DateString-Days.vi"("First date"=w272, "Second date"=w273) -> ("Elapsed days"=w270:i32)  [unwired: 8 in, 1 out]
            }
            frame 8 {
              n130 = Get Date/Time In Seconds() -> (seconds since 1Jan1904=w280:timestamp)
              n131 = Get Date/Time String(seconds (now)=w280) -> (date string=w278:string)  [unwired: 2 in, 1 out]
              n132 = Unbundle By Name(w281) -> ("Eq9"=w277:timestamp)
              n133 = Get Date/Time String(seconds (now)=w277) -> (date string=w279:string)  [unwired: 2 in, 1 out]
              n134 = call "DateString-Days.vi"("First date"=w278, "Second date"=w279) -> ("Elapsed days"=w276:i32)  [unwired: 8 in, 1 out]
            }
            frame 9 {
              n135 = Get Date/Time In Seconds() -> (seconds since 1Jan1904=w286:timestamp)
              n136 = Get Date/Time String(seconds (now)=w286) -> (date string=w284:string)  [unwired: 2 in, 1 out]
              n137 = Unbundle By Name(w287) -> ("Eq10"=w283:timestamp)
              n138 = Get Date/Time String(seconds (now)=w283) -> (date string=w285:string)  [unwired: 2 in, 1 out]
              n139 = call "DateString-Days.vi"("First date"=w284, "Second date"=w285) -> ("Elapsed days"=w282:i32)  [unwired: 8 in, 1 out]
            }
            frame 10 {
              n140 = Get Date/Time In Seconds() -> (seconds since 1Jan1904=w292:timestamp)
              n141 = Unbundle By Name(w293) -> ("Eq11"=w289:timestamp)
              n142 = Get Date/Time String(seconds (now)=w292) -> (date string=w290:string)  [unwired: 2 in, 1 out]
              n143 = Get Date/Time String(seconds (now)=w289) -> (date string=w291:string)  [unwired: 2 in, 1 out]
              n144 = call "DateString-Days.vi"("First date"=w290, "Second date"=w291) -> ("Elapsed days"=w288:i32)  [unwired: 8 in, 1 out]
            }
            frame 11 {
              n145 = Get Date/Time In Seconds() -> (seconds since 1Jan1904=w298:timestamp)
              n146 = Unbundle By Name(w299) -> ("Eq12"=w295:timestamp)
              n147 = Get Date/Time String(seconds (now)=w298) -> (date string=w296:string)  [unwired: 2 in, 1 out]
              n148 = Get Date/Time String(seconds (now)=w295) -> (date string=w297:string)  [unwired: 2 in, 1 out]
              n149 = call "DateString-Days.vi"("First date"=w296, "Second date"=w297) -> ("Elapsed days"=w294:i32)  [unwired: 8 in, 1 out]
            }
            frame 12 {
              n150 = Get Date/Time In Seconds() -> (seconds since 1Jan1904=w304:timestamp)
              n151 = Unbundle By Name(w305) -> ("Eq13"=w301:timestamp)
              n152 = Get Date/Time String(seconds (now)=w304) -> (date string=w302:string)  [unwired: 2 in, 1 out]
              n153 = Get Date/Time String(seconds (now)=w301) -> (date string=w303:string)  [unwired: 2 in, 1 out]
              n154 = call "DateString-Days.vi"("First date"=w302, "Second date"=w303) -> ("Elapsed days"=w300:i32)  [unwired: 8 in, 1 out]
            }
            frame 13 {
              n155 = Get Date/Time In Seconds() -> (seconds since 1Jan1904=w310:timestamp)
              n156 = Unbundle By Name(w311) -> ("Eq14"=w307:timestamp)
              n157 = Get Date/Time String(seconds (now)=w310) -> (date string=w308:string)  [unwired: 2 in, 1 out]
              n158 = Get Date/Time String(seconds (now)=w307) -> (date string=w309:string)  [unwired: 2 in, 1 out]
              n159 = call "DateString-Days.vi"("First date"=w308, "Second date"=w309) -> ("Elapsed days"=w306:i32)  [unwired: 8 in, 1 out]
            }
            frame 14 {
              n160 = Get Date/Time In Seconds() -> (seconds since 1Jan1904=w316:timestamp)
              n161 = Get Date/Time String(seconds (now)=w316) -> (date string=w314:string)  [unwired: 2 in, 1 out]
              n162 = Unbundle By Name(w317) -> ("Eq15"=w313:timestamp)
              n163 = Get Date/Time String(seconds (now)=w313) -> (date string=w315:string)  [unwired: 2 in, 1 out]
              n164 = call "DateString-Days.vi"("First date"=w314, "Second date"=w315) -> ("Elapsed days"=w312:i32)  [unwired: 8 in, 1 out]
            }
            frame 15 {
              n165 = Get Date/Time In Seconds() -> (seconds since 1Jan1904=w322:timestamp)
              n166 = Unbundle By Name(w323) -> ("Eq16"=w319:timestamp)
              n167 = Get Date/Time String(seconds (now)=w322) -> (date string=w320:string)  [unwired: 2 in, 1 out]
              n168 = Get Date/Time String(seconds (now)=w319) -> (date string=w321:string)  [unwired: 2 in, 1 out]
              n169 = call "DateString-Days.vi"("First date"=w320, "Second date"=w321) -> ("Elapsed days"=w318:i32)  [unwired: 8 in, 1 out]
            }
            frame 16 {
              n170 = Get Date/Time In Seconds() -> (seconds since 1Jan1904=w328:timestamp)
              n171 = Unbundle By Name(w329) -> ("Eq17"=w325:timestamp)
              n172 = Get Date/Time String(seconds (now)=w328) -> (date string=w326:string)  [unwired: 2 in, 1 out]
              n173 = Get Date/Time String(seconds (now)=w325) -> (date string=w327:string)  [unwired: 2 in, 1 out]
              n174 = call "DateString-Days.vi"("First date"=w326, "Second date"=w327) -> ("Elapsed days"=w324:i32)  [unwired: 8 in, 1 out]
            }
            frame 17 {
              n175 = Unbundle By Name(w335) -> ("Eq18"=w331:timestamp)
              n176 = Get Date/Time In Seconds() -> (seconds since 1Jan1904=w334:timestamp)
              n177 = Get Date/Time String(seconds (now)=w334) -> (date string=w332:string)  [unwired: 2 in, 1 out]
              n178 = Get Date/Time String(seconds (now)=w331) -> (date string=w333:string)  [unwired: 2 in, 1 out]
              n179 = call "DateString-Days.vi"("First date"=w332, "Second date"=w333) -> ("Elapsed days"=w330:i32)  [unwired: 8 in, 1 out]
            }
            frame 18 {
              n180 = Get Date/Time In Seconds() -> (seconds since 1Jan1904=w340:timestamp)
              n181 = Unbundle By Name(w341) -> ("Eq19"=w337:timestamp)
              n182 = Get Date/Time String(seconds (now)=w340) -> (date string=w338:string)  [unwired: 2 in, 1 out]
              n183 = Get Date/Time String(seconds (now)=w337) -> (date string=w339:string)  [unwired: 2 in, 1 out]
              n184 = call "DateString-Days.vi"("First date"=w338, "Second date"=w339) -> ("Elapsed days"=w336:i32)  [unwired: 8 in, 1 out]
            }
            frame 19 {
              n185 = Get Date/Time In Seconds() -> (seconds since 1Jan1904=w346:timestamp)
              n186 = Unbundle By Name(w347) -> ("Eq20"=w343:timestamp)
              n187 = Get Date/Time String(seconds (now)=w346) -> (date string=w344:string)  [unwired: 2 in, 1 out]
              n188 = Get Date/Time String(seconds (now)=w343) -> (date string=w345:string)  [unwired: 2 in, 1 out]
              n189 = call "DateString-Days.vi"("First date"=w344, "Second date"=w345) -> ("Elapsed days"=w342:i32)  [unwired: 8 in, 1 out]
            }
          }
        }
        n190 = Array Max & Min(array=w214) -> (min value=w211:i32)  [unwired: 3 out]
        n191 = Less?(x=w211, y=30) -> (x < y?=w212:bool)
        n192 = Number To Decimal String(number=w211) -> (decimal integer string=w210:string)  [unwired: 1 in]
        n193 = case shown="True" w212 {
          tunnel: w210 -> [_ w224]
          frame False {
          }
          frame True {
            n194 = Concatenate Strings("Componets will be out of calibration in " ("message"), w224, " Days" ("string")) -> (→"concatenated string":string)
          }
        }
        n195 = call <vilib>:"Add State(s) to Queue__jki_lib_state_machine.vi"("State(s) in (\"\")"=w220) -> ("States Out"=w219:string)  [unwired: 14 in]
      }
      frame "Equipment Desc" {
        # "Your code here.\n(You can make a copy of, or modify, this frame)"
        n196 = Unbundle By Name(w355) -> ("Equipment Description"=w353:T1, "Total Array"=w352:string[][])
        n197 = for {
          N: 20 -> [_]
          tunnel: w353 -> [w367]
          tunnel: string[] [] -> [w365]
          tunnel: [w364] -> w350 mode=indexing
          tunnel: [w363] -> w356
          tunnel: w357 -> [w363]
          i -> [w366]
          n198 = case shown="15" w366 {
            tunnel: w367 -> [w369 w371 w373 w375 w377 w379 w381 w383 w385 w387 w389 w391 w393 w395 w397 w399 w401 w402 w405 w407]
            tunnel: [w368 w370 w372 w374 w376 w378 w380 w382 w384 w386 w388 w390 w392 w394 w396 w398 w400 w403 w404 w406] -> w362
            frame 0, Default {
              n199 = Unbundle By Name(w369) -> ("Eq1"=w368:string)
            }
            frame 1 {
              n200 = Unbundle By Name(w371) -> ("Eq2"=w370:string)
            }
            frame 2 {
              n201 = Unbundle By Name(w373) -> ("Eq3"=w372:string)
            }
            frame 3 {
              n202 = Unbundle By Name(w375) -> ("Eq4"=w374:string)
            }
            frame 4 {
              n203 = Unbundle By Name(w377) -> ("Eq5"=w376:string)
            }
            frame 5 {
              n204 = Unbundle By Name(w379) -> ("Eq6"=w378:string)
            }
            frame 6 {
              n205 = Unbundle By Name(w381) -> ("Eq7"=w380:string)
            }
            frame 7 {
              n206 = Unbundle By Name(w383) -> ("Eq8"=w382:string)
            }
            frame 8 {
              n207 = Unbundle By Name(w385) -> ("Eq9"=w384:string)
            }
            frame 9 {
              n208 = Unbundle By Name(w387) -> ("Eq10"=w386:string)
            }
            frame 10 {
              n209 = Unbundle By Name(w389) -> ("Eq11"=w388:string)
            }
            frame 11 {
              n210 = Unbundle By Name(w391) -> ("Eq12"=w390:string)
            }
            frame 12 {
              n211 = Unbundle By Name(w393) -> ("Eq13"=w392:string)
            }
            frame 13 {
              n212 = Unbundle By Name(w395) -> ("Eq14"=w394:string)
            }
            frame 14 {
              n213 = Unbundle By Name(w397) -> ("Eq15"=w396:string)
            }
            frame 15 {
              n214 = Unbundle By Name(w399) -> ("Eq16"=w398:string)
            }
            frame 16 {
              n215 = Unbundle By Name(w401) -> ("Eq17"=w400:string)
            }
            frame 17 {
              n216 = Unbundle By Name(w402) -> ("Eq18"=w403:string)
            }
            frame 18 {
              n217 = Unbundle By Name(w405) -> ("Eq19"=w404:string)
            }
            frame 19 {
              n218 = Unbundle By Name(w407) -> ("Eq20"=w406:string)
            }
          }
          n219 = Build Array (concatenate)(w365, w362) -> (w364:string[])
        }
        n220 = call "Array-Get 1D str Column fr 2D.vi"("2D Array Data"=w350, "column index"=0) -> ("Column Data"=w348:string[])  [unwired: 13 in]
        n221 = Build Array (concatenate)(w352, w348) -> (w351:string[][])
        n222 = Bundle By Name(cluster=w355, "Total Array"=w351) -> (w354:T7)
        n223 = call <vilib>:"Add State(s) to Queue__jki_lib_state_machine.vi"("State(s) in (\"\")"=w361) -> ("States Out"=w360:string)  [unwired: 14 in]
      }
      frame "Manufacturer" {
        # "Your code here.\n(You can make a copy of, or modify, this frame)"
        n224 = Unbundle By Name(w415) -> ("Manufacturer"=w413:T1, "Total Array"=w412:string[][])
        n225 = for {
          N: 20 -> [_]
          tunnel: w413 -> [w427]
          tunnel: string[] [] -> [w425]
          tunnel: [w424] -> w410 mode=indexing
          tunnel: [w423] -> w416
          tunnel: w417 -> [w423]
          i -> [w426]
          n226 = case shown="15" w426 {
            tunnel: w427 -> [w429 w431 w433 w435 w437 w439 w441 w443 w445 w447 w449 w451 w453 w455 w457 w459 w461 w462 w465 w467]
            tunnel: [w428 w430 w432 w434 w436 w438 w440 w442 w444 w446 w448 w450 w452 w454 w456 w458 w460 w463 w464 w466] -> w422
            frame 0, Default {
              n227 = Unbundle By Name(w429) -> ("Eq1"=w428:string)
            }
            frame 1 {
              n228 = Unbundle By Name(w431) -> ("Eq2"=w430:string)
            }
            frame 2 {
              n229 = Unbundle By Name(w433) -> ("Eq3"=w432:string)
            }
            frame 3 {
              n230 = Unbundle By Name(w435) -> ("Eq4"=w434:string)
            }
            frame 4 {
              n231 = Unbundle By Name(w437) -> ("Eq5"=w436:string)
            }
            frame 5 {
              n232 = Unbundle By Name(w439) -> ("Eq6"=w438:string)
            }
            frame 6 {
              n233 = Unbundle By Name(w441) -> ("Eq7"=w440:string)
            }
            frame 7 {
              n234 = Unbundle By Name(w443) -> ("Eq8"=w442:string)
            }
            frame 8 {
              n235 = Unbundle By Name(w445) -> ("Eq9"=w444:string)
            }
            frame 9 {
              n236 = Unbundle By Name(w447) -> ("Eq10"=w446:string)
            }
            frame 10 {
              n237 = Unbundle By Name(w449) -> ("Eq11"=w448:string)
            }
            frame 11 {
              n238 = Unbundle By Name(w451) -> ("Eq12"=w450:string)
            }
            frame 12 {
              n239 = Unbundle By Name(w453) -> ("Eq13"=w452:string)
            }
            frame 13 {
              n240 = Unbundle By Name(w455) -> ("Eq14"=w454:string)
            }
            frame 14 {
              n241 = Unbundle By Name(w457) -> ("Eq15"=w456:string)
            }
            frame 15 {
              n242 = Unbundle By Name(w459) -> ("Eq16"=w458:string)
            }
            frame 16 {
              n243 = Unbundle By Name(w461) -> ("Eq17"=w460:string)
            }
            frame 17 {
              n244 = Unbundle By Name(w462) -> ("Eq18"=w463:string)
            }
            frame 18 {
              n245 = Unbundle By Name(w465) -> ("Eq19"=w464:string)
            }
            frame 19 {
              n246 = Unbundle By Name(w467) -> ("Eq20"=w466:string)
            }
          }
          n247 = Build Array (concatenate)(w425, w422) -> (w424:string[])
        }
        n248 = call "Array-Get 1D str Column fr 2D.vi"("2D Array Data"=w410, "column index"=0) -> ("Column Data"=w408:string[])  [unwired: 13 in]
        n249 = Build Array (concatenate)(w412, w408) -> (w411:string[][])
        n250 = Bundle By Name(cluster=w415, "Total Array"=w411) -> (w414:T7)
        n251 = call <vilib>:"Add State(s) to Queue__jki_lib_state_machine.vi"("State(s) in (\"\")"=w421) -> ("States Out"=w420:string)  [unwired: 14 in]
      }
      frame "Model Number" {
        # "Your code here.\n(You can make a copy of, or modify, this frame)"
        n252 = Unbundle By Name(w475) -> ("Model Number"=w473:T1, "Total Array"=w472:string[][])
        n253 = for {
          N: 20 -> [_]
          tunnel: w473 -> [w487]
          tunnel: string[] [] -> [w485]
          tunnel: [w484] -> w470 mode=indexing
          tunnel: [w483] -> w476
          tunnel: w477 -> [w483]
          i -> [w486]
          n254 = case shown="15" w486 {
            tunnel: w487 -> [w489 w491 w493 w495 w497 w499 w501 w503 w505 w507 w509 w511 w513 w515 w517 w519 w521 w522 w525 w527]
            tunnel: [w488 w490 w492 w494 w496 w498 w500 w502 w504 w506 w508 w510 w512 w514 w516 w518 w520 w523 w524 w526] -> w482
            frame 0, Default {
              n255 = Unbundle By Name(w489) -> ("Eq1"=w488:string)
            }
            frame 1 {
              n256 = Unbundle By Name(w491) -> ("Eq2"=w490:string)
            }
            frame 2 {
              n257 = Unbundle By Name(w493) -> ("Eq3"=w492:string)
            }
            frame 3 {
              n258 = Unbundle By Name(w495) -> ("Eq4"=w494:string)
            }
            frame 4 {
              n259 = Unbundle By Name(w497) -> ("Eq5"=w496:string)
            }
            frame 5 {
              n260 = Unbundle By Name(w499) -> ("Eq6"=w498:string)
            }
            frame 6 {
              n261 = Unbundle By Name(w501) -> ("Eq7"=w500:string)
            }
            frame 7 {
              n262 = Unbundle By Name(w503) -> ("Eq8"=w502:string)
            }
            frame 8 {
              n263 = Unbundle By Name(w505) -> ("Eq9"=w504:string)
            }
            frame 9 {
              n264 = Unbundle By Name(w507) -> ("Eq10"=w506:string)
            }
            frame 10 {
              n265 = Unbundle By Name(w509) -> ("Eq11"=w508:string)
            }
            frame 11 {
              n266 = Unbundle By Name(w511) -> ("Eq12"=w510:string)
            }
            frame 12 {
              n267 = Unbundle By Name(w513) -> ("Eq13"=w512:string)
            }
            frame 13 {
              n268 = Unbundle By Name(w515) -> ("Eq14"=w514:string)
            }
            frame 14 {
              n269 = Unbundle By Name(w517) -> ("Eq15"=w516:string)
            }
            frame 15 {
              n270 = Unbundle By Name(w519) -> ("Eq16"=w518:string)
            }
            frame 16 {
              n271 = Unbundle By Name(w521) -> ("Eq17"=w520:string)
            }
            frame 17 {
              n272 = Unbundle By Name(w522) -> ("Eq18"=w523:string)
            }
            frame 18 {
              n273 = Unbundle By Name(w525) -> ("Eq19"=w524:string)
            }
            frame 19 {
              n274 = Unbundle By Name(w527) -> ("Eq20"=w526:string)
            }
          }
          n275 = Build Array (concatenate)(w485, w482) -> (w484:string[])
        }
        n276 = call "Array-Get 1D str Column fr 2D.vi"("2D Array Data"=w470, "column index"=0) -> ("Column Data"=w468:string[])  [unwired: 13 in]
        n277 = Build Array (concatenate)(w472, w468) -> (w471:string[][])
        n278 = Bundle By Name(cluster=w475, "Total Array"=w471) -> (w474:T7)
        n279 = call <vilib>:"Add State(s) to Queue__jki_lib_state_machine.vi"("State(s) in (\"\")"=w481) -> ("States Out"=w480:string)  [unwired: 14 in]
      }
      frame "Write Calibration ID" {
        # "Your code here.\n(You can make a copy of, or modify, this frame)"
        n280 = Unbundle By Name(w535) -> ("Calibration ID"=w533:T1, "Total Array"=w532:string[][])
        n281 = for {
          N: 20 -> [_]
          tunnel: w533 -> [w547]
          tunnel: string[] [] -> [w545]
          tunnel: [w544] -> w530 mode=indexing
          tunnel: [w543] -> w536
          tunnel: w537 -> [w543]
          i -> [w546]
          n282 = case shown="15" w546 {
            tunnel: w547 -> [w549 w551 w553 w555 w557 w559 w561 w563 w565 w567 w569 w571 w573 w575 w577 w579 w581 w582 w585 w587]
            tunnel: [w548 w550 w552 w554 w556 w558 w560 w562 w564 w566 w568 w570 w572 w574 w576 w578 w580 w583 w584 w586] -> w542
            frame 0, Default {
              n283 = Unbundle By Name(w549) -> ("Eq1"=w548:string)
            }
            frame 1 {
              n284 = Unbundle By Name(w551) -> ("Eq2"=w550:string)
            }
            frame 2 {
              n285 = Unbundle By Name(w553) -> ("Eq3"=w552:string)
            }
            frame 3 {
              n286 = Unbundle By Name(w555) -> ("Eq4"=w554:string)
            }
            frame 4 {
              n287 = Unbundle By Name(w557) -> ("Eq5"=w556:string)
            }
            frame 5 {
              n288 = Unbundle By Name(w559) -> ("Eq6"=w558:string)
            }
            frame 6 {
              n289 = Unbundle By Name(w561) -> ("Eq7"=w560:string)
            }
            frame 7 {
              n290 = Unbundle By Name(w563) -> ("Eq8"=w562:string)
            }
            frame 8 {
              n291 = Unbundle By Name(w565) -> ("Eq9"=w564:string)
            }
            frame 9 {
              n292 = Unbundle By Name(w567) -> ("Eq10"=w566:string)
            }
            frame 10 {
              n293 = Unbundle By Name(w569) -> ("Eq11"=w568:string)
            }
            frame 11 {
              n294 = Unbundle By Name(w571) -> ("Eq12"=w570:string)
            }
            frame 12 {
              n295 = Unbundle By Name(w573) -> ("Eq13"=w572:string)
            }
            frame 13 {
              n296 = Unbundle By Name(w575) -> ("Eq14"=w574:string)
            }
            frame 14 {
              n297 = Unbundle By Name(w577) -> ("Eq15"=w576:string)
            }
            frame 15 {
              n298 = Unbundle By Name(w579) -> ("Eq16"=w578:string)
            }
            frame 16 {
              n299 = Unbundle By Name(w581) -> ("Eq17"=w580:string)
            }
            frame 17 {
              n300 = Unbundle By Name(w582) -> ("Eq18"=w583:string)
            }
            frame 18 {
              n301 = Unbundle By Name(w585) -> ("Eq19"=w584:string)
            }
            frame 19 {
              n302 = Unbundle By Name(w587) -> ("Eq20"=w586:string)
            }
          }
          n303 = Build Array (concatenate)(w545, w542) -> (w544:string[])
        }
        n304 = call "Array-Get 1D str Column fr 2D.vi"("2D Array Data"=w530, "column index"=0) -> ("Column Data"=w528:string[])  [unwired: 13 in]
        n305 = Build Array (concatenate)(w532, w528) -> (w531:string[][])
        n306 = Bundle By Name(cluster=w535, "Total Array"=w531) -> (w534:T7)
        n307 = call <vilib>:"Add State(s) to Queue__jki_lib_state_machine.vi"("State(s) in (\"\")"=w541) -> ("States Out"=w540:string)  [unwired: 14 in]
      }
      frame "Write Calibration SN" {
        n308 = Unbundle By Name(w595) -> ("Serial Number"=w593:T2, "Total Array"=w592:string[][])
        n309 = for {
          N: 20 -> [_]
          tunnel: w593 -> [w607]
          tunnel: string[] [] -> [w605]
          tunnel: [w604] -> w590 mode=indexing
          tunnel: [w603] -> w596
          tunnel: w597 -> [w603]
          i -> [w606]
          n310 = case shown="15" w606 {
            tunnel: w607 -> [w609 w611 w613 w615 w617 w619 w621 w623 w625 w627 w629 w631 w633 w635 w637 w639 w641 w643 w645 w647]
            tunnel: [w608 w610 w612 w614 w616 w618 w620 w622 w624 w626 w628 w630 w632 w634 w636 w638 w640 w642 w644 w646] -> w602
            frame 0, Default {
              n311 = Unbundle By Name(w609) -> ("Eq1"=w608:string)
            }
            frame 1 {
              n312 = Unbundle By Name(w611) -> ("Eq2"=w610:string)
            }
            frame 2 {
              n313 = Unbundle By Name(w613) -> ("Eq3"=w612:string)
            }
            frame 3 {
              n314 = Unbundle By Name(w615) -> ("Eq4"=w614:string)
            }
            frame 4 {
              n315 = Unbundle By Name(w617) -> ("Eq5"=w616:string)
            }
            frame 5 {
              n316 = Unbundle By Name(w619) -> ("Eq6"=w618:string)
            }
            frame 6 {
              n317 = Unbundle By Name(w621) -> ("Eq7"=w620:string)
            }
            frame 7 {
              n318 = Unbundle By Name(w623) -> ("Eq8"=w622:string)
            }
            frame 8 {
              n319 = Unbundle By Name(w625) -> ("Eq9"=w624:string)
            }
            frame 9 {
              n320 = Unbundle By Name(w627) -> ("Eq10"=w626:string)
            }
            frame 10 {
              n321 = Unbundle By Name(w629) -> ("Eq11"=w628:string)
            }
            frame 11 {
              n322 = Unbundle By Name(w631) -> ("Eq12"=w630:string)
            }
            frame 12 {
              n323 = Unbundle By Name(w633) -> ("Eq13"=w632:string)
            }
            frame 13 {
              n324 = Unbundle By Name(w635) -> ("Eq14"=w634:string)
            }
            frame 14 {
              n325 = Unbundle By Name(w637) -> ("Eq15"=w636:string)
            }
            frame 15 {
              n326 = Unbundle By Name(w639) -> ("Eq16"=w638:string)
            }
            frame 16 {
              n327 = Unbundle By Name(w641) -> ("Eq17"=w640:string)
            }
            frame 17 {
              n328 = Unbundle By Name(w643) -> ("Eq18"=w642:string)
            }
            frame 18 {
              n329 = Unbundle By Name(w645) -> ("Eq19"=w644:string)
            }
            frame 19 {
              n330 = Unbundle By Name(w647) -> ("Eq20"=w646:string)
            }
          }
          n331 = Build Array (concatenate)(w605, w602) -> (w604:string[])
        }
        n332 = call "Array-Get 1D str Column fr 2D.vi"("2D Array Data"=w590, "column index"=0) -> ("Column Data"=w588:string[])  [unwired: 13 in]
        "snta" <- w588
        n333 = Build Array (concatenate)(w592, w588) -> (w591:string[][])
        n334 = Bundle By Name(cluster=w595, "Total Array"=w591) -> (w594:T7)
        n335 = call <vilib>:"Add State(s) to Queue__jki_lib_state_machine.vi"("State(s) in (\"\")"=w601) -> ("States Out"=w600:string)  [unwired: 14 in]
      }
      frame "Last Calibration" {
        n336 = Unbundle By Name(w654) -> ("Last Calibrated"=w655:T3, "Total Array"=w650:string[][])
        n337 = for {
          N: 20 -> [_]
          tunnel: w655 -> [w669]
          tunnel: string[] [] -> [w667]
          tunnel: [w666] -> w652 mode=indexing
          tunnel: [w662] -> w656
          tunnel: w657 -> [w662]
          i -> [w668]
          n338 = case shown="0, Default" w668 {
            tunnel: w669 -> [w672 w675 w678 w681 w684 w687 w690 w693 w696 w699 w702 w705 w708 w711 w714 w717 w720 w723 w725 w729]
            tunnel: [w670 w673 w676 w679 w682 w685 w688 w691 w694 w697 w700 w703 w706 w709 w712 w715 w718 w721 w726 w727] -> w665
            frame 0, Default {
              n339 = Unbundle By Name(w672) -> ("Eq1"=w671:timestamp)
              n340 = Format Date/Time String(seconds (now)=w671) -> (date/time string=w670:string)  [unwired: 2 in]
            }
            frame 1 {
              n341 = Unbundle By Name(w675) -> ("Eq2"=w674:timestamp)
              n342 = Format Date/Time String(seconds (now)=w674) -> (date/time string=w673:string)  [unwired: 2 in]
            }
            frame 2 {
              n343 = Unbundle By Name(w678) -> ("Eq3"=w677:timestamp)
              n344 = Format Date/Time String(seconds (now)=w677) -> (date/time string=w676:string)  [unwired: 2 in]
            }
            frame 3 {
              n345 = Unbundle By Name(w681) -> ("Eq4"=w680:timestamp)
              n346 = Format Date/Time String(seconds (now)=w680) -> (date/time string=w679:string)  [unwired: 2 in]
            }
            frame 4 {
              n347 = Unbundle By Name(w684) -> ("Eq5"=w683:timestamp)
              n348 = Format Date/Time String(seconds (now)=w683) -> (date/time string=w682:string)  [unwired: 2 in]
            }
            frame 5 {
              n349 = Unbundle By Name(w687) -> ("Eq6"=w686:timestamp)
              n350 = Format Date/Time String(seconds (now)=w686) -> (date/time string=w685:string)  [unwired: 2 in]
            }
            frame 6 {
              n351 = Unbundle By Name(w690) -> ("Eq7"=w689:timestamp)
              n352 = Format Date/Time String(seconds (now)=w689) -> (date/time string=w688:string)  [unwired: 2 in]
            }
            frame 7 {
              n353 = Unbundle By Name(w693) -> ("Eq8"=w692:timestamp)
              n354 = Format Date/Time String(seconds (now)=w692) -> (date/time string=w691:string)  [unwired: 2 in]
            }
            frame 8 {
              n355 = Unbundle By Name(w696) -> ("Eq9"=w695:timestamp)
              n356 = Format Date/Time String(seconds (now)=w695) -> (date/time string=w694:string)  [unwired: 2 in]
            }
            frame 9 {
              n357 = Unbundle By Name(w699) -> ("Eq10"=w698:timestamp)
              n358 = Format Date/Time String(seconds (now)=w698) -> (date/time string=w697:string)  [unwired: 2 in]
            }
            frame 10 {
              n359 = Unbundle By Name(w702) -> ("Eq11"=w701:timestamp)
              n360 = Format Date/Time String(seconds (now)=w701) -> (date/time string=w700:string)  [unwired: 2 in]
            }
            frame 11 {
              n361 = Unbundle By Name(w705) -> ("Eq12"=w704:timestamp)
              n362 = Format Date/Time String(seconds (now)=w704) -> (date/time string=w703:string)  [unwired: 2 in]
            }
            frame 12 {
              n363 = Unbundle By Name(w708) -> ("Eq13"=w707:timestamp)
              n364 = Format Date/Time String(seconds (now)=w707) -> (date/time string=w706:string)  [unwired: 2 in]
            }
            frame 13 {
              n365 = Unbundle By Name(w711) -> ("Eq14"=w710:timestamp)
              n366 = Format Date/Time String(seconds (now)=w710) -> (date/time string=w709:string)  [unwired: 2 in]
            }
            frame 14 {
              n367 = Unbundle By Name(w714) -> ("Eq15"=w713:timestamp)
              n368 = Format Date/Time String(seconds (now)=w713) -> (date/time string=w712:string)  [unwired: 2 in]
            }
            frame 15 {
              n369 = Unbundle By Name(w717) -> ("Eq16"=w716:timestamp)
              n370 = Format Date/Time String(seconds (now)=w716) -> (date/time string=w715:string)  [unwired: 2 in]
            }
            frame 16 {
              n371 = Unbundle By Name(w720) -> ("Eq17"=w719:timestamp)
              n372 = Format Date/Time String(seconds (now)=w719) -> (date/time string=w718:string)  [unwired: 2 in]
            }
            frame 17 {
              n373 = Unbundle By Name(w723) -> ("Eq18"=w722:timestamp)
              n374 = Format Date/Time String(seconds (now)=w722) -> (date/time string=w721:string)  [unwired: 2 in]
            }
            frame 18 {
              n375 = Unbundle By Name(w725) -> ("Eq19"=w724:timestamp)
              n376 = Format Date/Time String(seconds (now)=w724) -> (date/time string=w726:string)  [unwired: 2 in]
            }
            frame 19 {
              n377 = Unbundle By Name(w729) -> ("Eq20"=w728:timestamp)
              n378 = Format Date/Time String(seconds (now)=w728) -> (date/time string=w727:string)  [unwired: 2 in]
            }
          }
          n379 = call <vilib>:"Space Constant.vi"() -> ("String"=w663:string)
          n380 = Match Pattern(string=w665, regular expression=w663) -> (before substring=w664:string)  [unwired: 1 in, 3 out]
          n381 = Build Array (concatenate)(w667, w664) -> (w666:string[])
        }
        n382 = call "Array-Get 1D str Column fr 2D.vi"("2D Array Data"=w652, "column index"=0) -> ("Column Data"=w649:string[])  [unwired: 13 in]
        n383 = Build Array (concatenate)(w650, w649) -> (w648:string[][])
        n384 = Bundle By Name(cluster=w654, "Total Array"=w648) -> (w653:T7)
        n385 = call <vilib>:"Add State(s) to Queue__jki_lib_state_machine.vi"("State(s) in (\"\")"=w661) -> ("States Out"=w660:string)  [unwired: 14 in]
      }
      frame "Write Calibration Date" {
        n386 = Unbundle By Name(w736) -> ("Calibration Due"=w737:T3, "Total Array"=w732:string[][])
        n387 = for {
          N: 20 -> [_]
          tunnel: w737 -> [w751]
          tunnel: string[] [] -> [w749]
          tunnel: [w748] -> w734 mode=indexing
          tunnel: [w744] -> w738
          tunnel: w739 -> [w744]
          i -> [w750]
          n388 = case shown="15" w750 {
            tunnel: w751 -> [w754 w757 w760 w763 w766 w769 w772 w775 w778 w781 w784 w787 w790 w793 w796 w799 w802 w805 w807 w811]
            tunnel: [w752 w755 w758 w761 w764 w767 w770 w773 w776 w779 w782 w785 w788 w791 w794 w797 w800 w803 w808 w809] -> w747
            frame 0, Default {
              n389 = Unbundle By Name(w754) -> ("Eq1"=w753:timestamp)
              n390 = Format Date/Time String(seconds (now)=w753) -> (date/time string=w752:string)  [unwired: 2 in]
            }
            frame 1 {
              n391 = Unbundle By Name(w757) -> ("Eq2"=w756:timestamp)
              n392 = Format Date/Time String(seconds (now)=w756) -> (date/time string=w755:string)  [unwired: 2 in]
            }
            frame 2 {
              n393 = Unbundle By Name(w760) -> ("Eq3"=w759:timestamp)
              n394 = Format Date/Time String(seconds (now)=w759) -> (date/time string=w758:string)  [unwired: 2 in]
            }
            frame 3 {
              n395 = Unbundle By Name(w763) -> ("Eq4"=w762:timestamp)
              n396 = Format Date/Time String(seconds (now)=w762) -> (date/time string=w761:string)  [unwired: 2 in]
            }
            frame 4 {
              n397 = Unbundle By Name(w766) -> ("Eq5"=w765:timestamp)
              n398 = Format Date/Time String(seconds (now)=w765) -> (date/time string=w764:string)  [unwired: 2 in]
            }
            frame 5 {
              n399 = Unbundle By Name(w769) -> ("Eq6"=w768:timestamp)
              n400 = Format Date/Time String(seconds (now)=w768) -> (date/time string=w767:string)  [unwired: 2 in]
            }
            frame 6 {
              n401 = Unbundle By Name(w772) -> ("Eq7"=w771:timestamp)
              n402 = Format Date/Time String(seconds (now)=w771) -> (date/time string=w770:string)  [unwired: 2 in]
            }
            frame 7 {
              n403 = Unbundle By Name(w775) -> ("Eq8"=w774:timestamp)
              n404 = Format Date/Time String(seconds (now)=w774) -> (date/time string=w773:string)  [unwired: 2 in]
            }
            frame 8 {
              n405 = Unbundle By Name(w778) -> ("Eq9"=w777:timestamp)
              n406 = Format Date/Time String(seconds (now)=w777) -> (date/time string=w776:string)  [unwired: 2 in]
            }
            frame 9 {
              n407 = Unbundle By Name(w781) -> ("Eq10"=w780:timestamp)
              n408 = Format Date/Time String(seconds (now)=w780) -> (date/time string=w779:string)  [unwired: 2 in]
            }
            frame 10 {
              n409 = Unbundle By Name(w784) -> ("Eq11"=w783:timestamp)
              n410 = Format Date/Time String(seconds (now)=w783) -> (date/time string=w782:string)  [unwired: 2 in]
            }
            frame 11 {
              n411 = Unbundle By Name(w787) -> ("Eq12"=w786:timestamp)
              n412 = Format Date/Time String(seconds (now)=w786) -> (date/time string=w785:string)  [unwired: 2 in]
            }
            frame 12 {
              n413 = Unbundle By Name(w790) -> ("Eq13"=w789:timestamp)
              n414 = Format Date/Time String(seconds (now)=w789) -> (date/time string=w788:string)  [unwired: 2 in]
            }
            frame 13 {
              n415 = Unbundle By Name(w793) -> ("Eq14"=w792:timestamp)
              n416 = Format Date/Time String(seconds (now)=w792) -> (date/time string=w791:string)  [unwired: 2 in]
            }
            frame 14 {
              n417 = Unbundle By Name(w796) -> ("Eq15"=w795:timestamp)
              n418 = Format Date/Time String(seconds (now)=w795) -> (date/time string=w794:string)  [unwired: 2 in]
            }
            frame 15 {
              n419 = Unbundle By Name(w799) -> ("Eq16"=w798:timestamp)
              n420 = Format Date/Time String(seconds (now)=w798) -> (date/time string=w797:string)  [unwired: 2 in]
            }
            frame 16 {
              n421 = Unbundle By Name(w802) -> ("Eq17"=w801:timestamp)
              n422 = Format Date/Time String(seconds (now)=w801) -> (date/time string=w800:string)  [unwired: 2 in]
            }
            frame 17 {
              n423 = Unbundle By Name(w805) -> ("Eq18"=w804:timestamp)
              n424 = Format Date/Time String(seconds (now)=w804) -> (date/time string=w803:string)  [unwired: 2 in]
            }
            frame 18 {
              n425 = Unbundle By Name(w807) -> ("Eq19"=w806:timestamp)
              n426 = Format Date/Time String(seconds (now)=w806) -> (date/time string=w808:string)  [unwired: 2 in]
            }
            frame 19 {
              n427 = Unbundle By Name(w811) -> ("Eq20"=w810:timestamp)
              n428 = Format Date/Time String(seconds (now)=w810) -> (date/time string=w809:string)  [unwired: 2 in]
            }
          }
          n429 = call <vilib>:"Space Constant.vi"() -> ("String"=w745:string)
          n430 = Match Pattern(string=w747, regular expression=w745) -> (before substring=w746:string)  [unwired: 1 in, 3 out]
          n431 = Build Array (concatenate)(w749, w746) -> (w748:string[])
        }
        n432 = call "Array-Get 1D str Column fr 2D.vi"("2D Array Data"=w734, "column index"=0) -> ("Column Data"=w731:string[])  [unwired: 13 in]
        n433 = Build Array (concatenate)(w732, w731) -> (w730:string[][])
        n434 = Bundle By Name(cluster=w736, "Total Array"=w730) -> (w735:T7)
        n435 = call <vilib>:"Add State(s) to Queue__jki_lib_state_machine.vi"("State(s) in (\"\")"=w743) -> ("States Out"=w742:string)  [unwired: 14 in]
      }
      frame "Write to File" {
        # "Your code here.\n(You can make a copy of, or modify, this frame)"
        n436 = Unbundle By Name(w817) -> ("file path (dialog if empty)"=w816:path, "Total Array"=w812:string[][])
        n437 = Transpose 2D Array(2D array=w812) -> (transposed array=w813:string[][])
        "OutputData" <- w813
        n438 = call-poly <vilib>:"Write To Spreadsheet File.vi"("delimiter (\\t)"="," ("delimiter (\\t)"), "2D data"=w813, "file path (dialog if empty)"=w816) -> ()  [unwired: 5 in, 1 out]
        n439 = call <vilib>:"Add State(s) to Queue__jki_lib_state_machine.vi"("State(s) in (\"\")"=w819) -> ("States Out"=w818:string)  [unwired: 14 in]
      }
    }
  }
  "error out" <- w2
